vi "Get Command and Process.vi"(8 "Error In":errorcluster, 10 "FPGA Ref":T3, 11 "Network Info":T1 {"Last Comm Time" format="%<%H:%M:%S%3u\n%Y/%m/%d>T"; "Remote Port" format="%.0x"}) -> (0 "Error Out":errorcluster, 2 "Connection Dormant":bool, 3 "Network Info out":T1 {"Last Comm Time" format="%<%H:%M:%S%3u\n%Y/%m/%d>T"; "Remote Port" format="%.0x"})   [LabVIEW 2020]
doc: "Author: Scott Hannahs <sth@magnet.fsu.edu>\nCopyright 2018 Florida State University, All rights reserved."
uses:
  RT Controls/Network Info.ctl
  RT Controls/RT System Auth Level.ctl
  RT Controls/FPGA SCH Digitizer Ref.ctl
  Init Coil Calibration/FPGA Magnet Config.ctl
  SCH Data Controls/SCH Data 2 RT.ctl
  RT Host Globals.vi
  TCP Functions/TCP Write Length and Data (STR).vi
  TCP Functions/TCP Write Length and Data (DBL).vi
  TCP Functions/TCP Write Length and Data (2D Array DBL).vi
  TCP Functions/TCP Read Length and Value (STR).vi
  TCP Functions/TCP Read Length and Value (Array Dbl).vi
  <vilib>/Utility/error.llb/Error Cluster From Error Code.vi
  <vilib>/rvi/errors/niLvFpgaAdjustHostInterfaceError.vi
  TCP Functions/TCP Read Length and Value (Double).vi
  TCP Functions/TCP Read Length and Value (U32).vi
  TCP Functions/TCP Read Length and Value (I16).vi
  TCP Functions/TCP Read Length and Value (Bool).vi
  TCP Functions/TCP Read Length and Value (I32).vi
  TCP Functions/TCP Read Length and Value (U16).vi
  TCP Functions/TCP Write Length and Data (Array DBL).vi
  TCP Functions/TCP Write Length and Data (U32).vi
  TCP Functions/TCP Write Length and Data (Bool).vi
  TCP Functions/TCP Write Length and Data (I16).vi
  TCP Functions/TCP Write Length and Data (I32).vi
  TCP Functions/TCP Write Length and Data (Array I16).vi
  TCP Functions/TCP Write Length and Data (U16).vi
  TCP Functions/TCP Write Length and Data (DateStamp).vi
  TCP Functions/TCP Write Length and Data (Array Str).vi
  <vilib>/rvi/interface/nirviReadWriteControl/nirviReadWriteControl.xnode
  NiFpgaLv.dll
  <vilib>/rvi/interface/Simulation/niFpgaSimulationCallBeginRW.vi
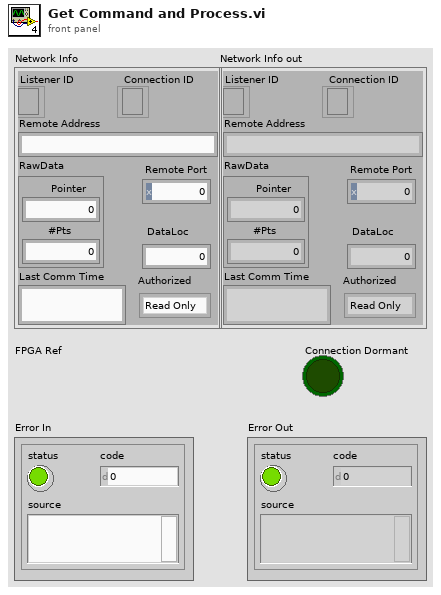
[diagram p1: front panel]
types:
  T1 = typedef "Network Info.ctl" = cluster{"Listener ID":refnum<k5>, "Connection ID":refnum<k5>, "Remote Address":string, "Remote Port":u16, "DataLoc":u32, "RawData":cluster{"#Pts":u32, "Pointer":u32}, "Last Comm Time":timestamp, "Authorized":T2}
  T2 = typedef "RT System Auth Level.ctl" = enum16{"Read Only", "Operator", "Admin"}
  T3 = typedef "FPGA SCH Digitizer Ref.ctl" = refnum<k20>
  T4 = typedef "FPGA Magnet Config.ctl" = cluster{"#Coils":u32, "Coil Inductances":T5[], "Max Coil Currents":T5[], "Max Coil Volt Dev":T5[], "Coil A Coefficients":T5[], "Coil B Coefficients":T5[], "Coil C Coefficients":T5[], "Coil D Coefficients":T5[], "Max Coil Temp":T5[], " Pressure Range":T5[], "Temp Coef":T5[], "Offsets":T5[], "Scale Factors":T5[]}
  T5 = typedef "SCH Data 2 RT.ctl" = fxp<+/-,38,12>
  T6 = enum16{"Input Voltage", "Zero Voltage", "Calibrate Voltage"}
  T7 = typedef "FPGA Configure Parameters.ctl" = cluster{"Ln2 Filter Size":i16, "VT Quench Tick Limit":u32, "VT Quench Volt Limit":dbl, "Joint Tick Limit":u32, "Joint Volt Limit":dbl, "CoWound Volt Limit":dbl, "CoWound Tick Limit":u32, "SC Bus Limit":dbl, "SC Bus Tick Limit":u32, "ResMag Tick Limit":u32, "DAQ Cycle Ticks":u32, "Res Mag dI/dt Delay":u32, "dI/dT scaling":dbl, "Pressure Inlet Limit (BarA)":dbl, "Bore Tube Volt Limit":dbl, "Pressure Outlet Limit (BarA)":dbl, "Activation Current (kA)":dbl, "Dump Resistor Scale Factor":dbl, "Co-Wound Asymmetry Factor":dbl, "Co-Wound Scale Factor":dbl, "Layer Scale Factors":dbl[], "Fudge Factors":dbl[], "Joint Scale Factors":dbl[], "SC Bus Scale":dbl[], "Pressure Scale Factor":dbl[], "# Consecutive Zeros Fault":i16, "Digitize Convert Ticks":u32, "Digitize Reset Ticks":u32, "Convert Clock Ticks":u32, "Digitize Read Delay Ticks":u32, "Digitize # Bits":u32, "HTS Lead Tick Limit":u32, "Res Lead Tick Limit":u32, "HTS Lead Trip":dbl, "Res Lead Limit":dbl, "HTS Lead FRZ":dbl, "HTS Lead Warn":dbl, "Low Current (kA)":dbl, "Low Current Ticks":u32, "Low Current Delay Factor":u16, "HTS Resistance (nOhm)":dbl[], "Ticks to Close Relief":u32, "All Breaker Tick Limit":u32, "HTS Offset (microV)":dbl[], "Delay Ticks Between Bkr Reset":u32, "Breaker Reset Ticks":u32, "PS Enable Reset Ticks":u32, "Reset Digitizer Ticks":u32, "Pressure Inlet Cooldown Limit":dbl, "Pressure Outlet Cooldown Limit":dbl, "Notification Email":string}
  T8 = cluster{"#Coils":u32, "Coil Inductances":fxp<+/-,38,12>[], "Max Coil Currents":fxp<+/-,38,12>[], "Max Coil Volt Dev":fxp<+/-,38,12>[], "Coil A Coefficients":fxp<+/-,38,12>[], "Coil B Coefficients":fxp<+/-,38,12>[], "Coil C Coefficients":fxp<+/-,38,12>[], "Coil D Coefficients":fxp<+/-,38,12>[], "Max Coil Temp":fxp<+/-,38,12>[], " Pressure Range":fxp<+/-,38,12>[], "Temp Coef":fxp<+/-,38,12>[], "Offsets":fxp<+/-,38,12>[], "Scale Factors":fxp<+/-,38,12>[]}
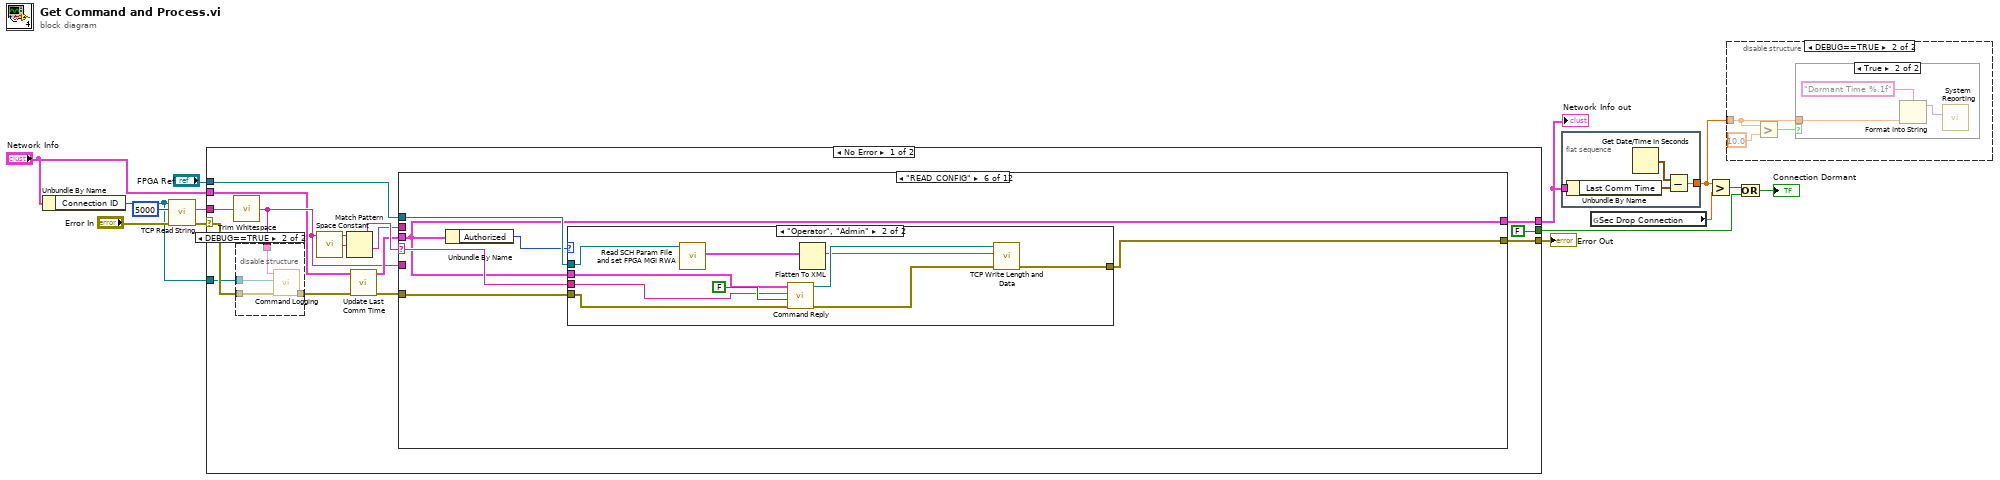
[diagram p0: block diagram]
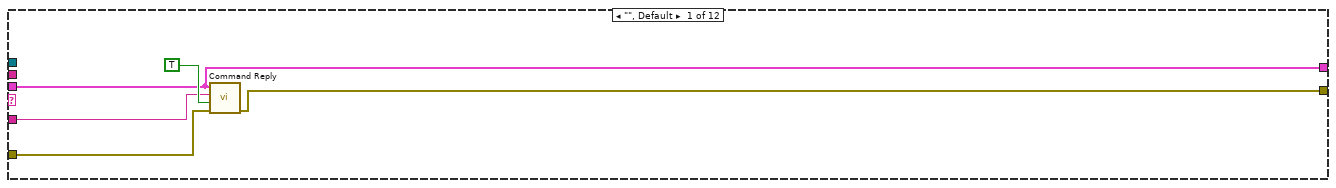
[diagram p5: hidden frame]
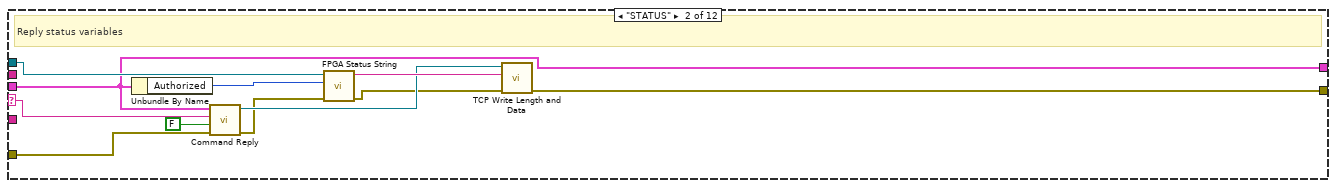
[diagram p6: hidden frame]
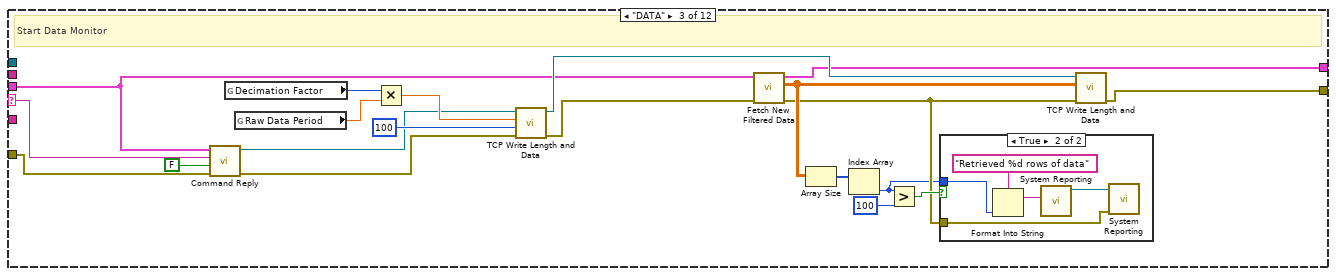
[diagram p7: hidden frame]
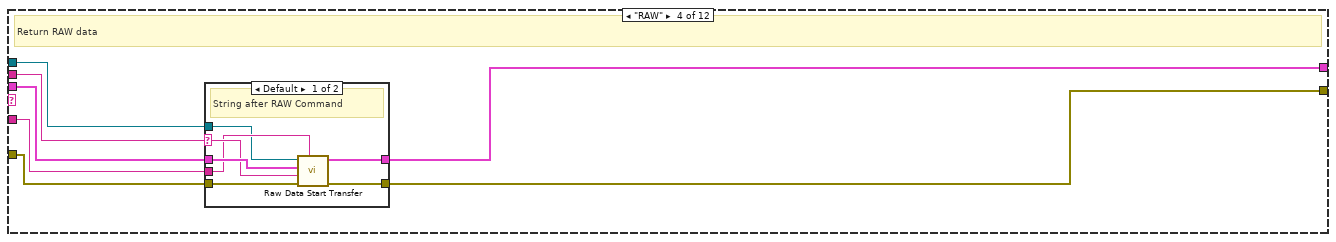
[diagram p9: hidden frame]
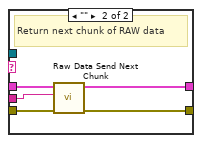
[diagram p10: hidden frame]
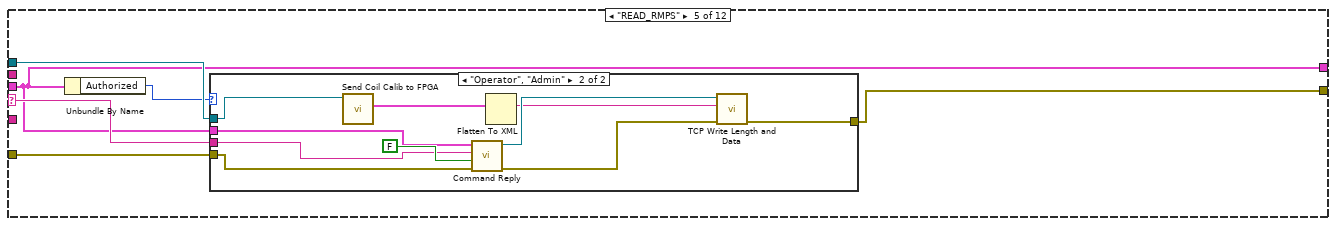
[diagram p11: hidden frame]
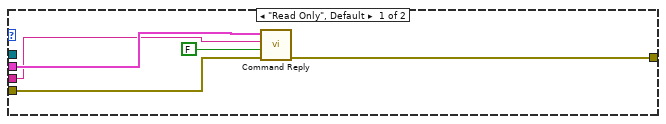
[diagram p12: hidden frame]
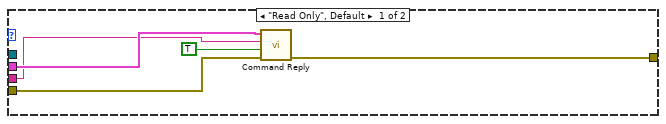
[diagram p13: hidden frame]
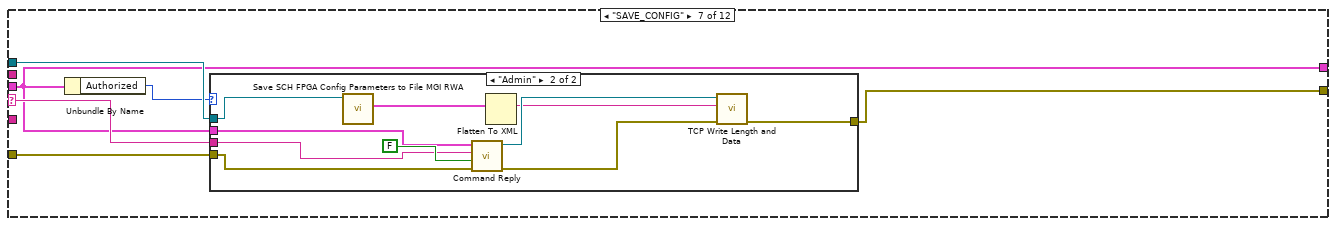
[diagram p14: hidden frame]
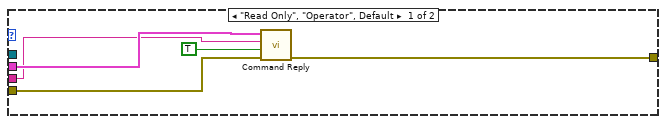
[diagram p15: hidden frame]
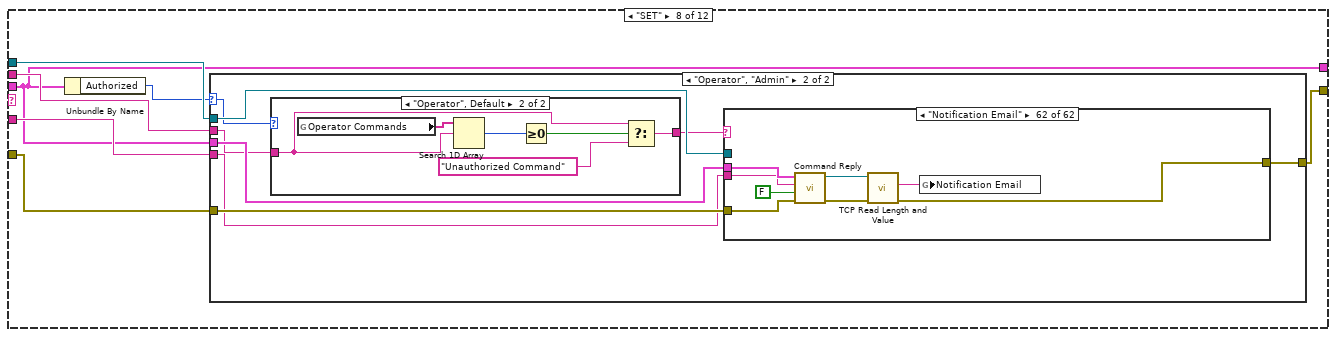
[diagram p16: hidden frame]
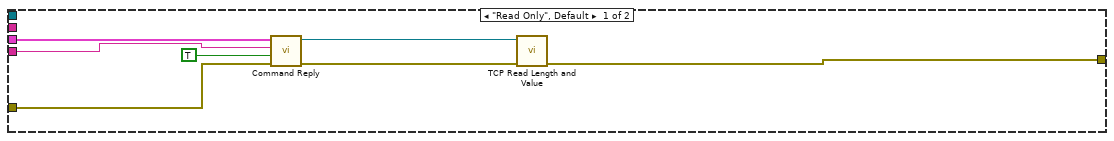
[diagram p17: hidden frame]
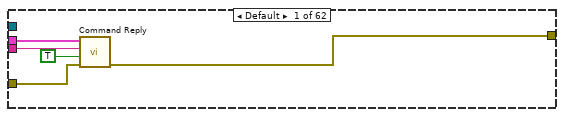
[diagram p19: hidden frame]
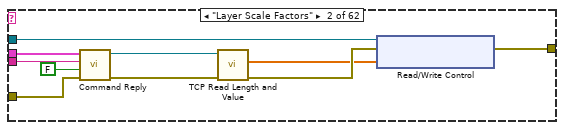
[diagram p20: hidden frame]
diagram:
  n1 = Unbundle By Name("Network Info") -> ("Connection ID"=w3:refnum<k5>)
  n2 = call "TCP Read String.vi"("Error In"="Error In", "timeout ms (1000)"=5000 ("timeout ms (25000)"), "TCP Network Connection in"=w3) -> ("Error Out"=w11:errorcluster, "String"=w9:string)  [unwired: 6 in, 1 out]
  n3 = case shown="No Error" w11 {
    selector: w11 -> [w21 w1545]
    tunnel: "Network Info" -> [w16 w1547]
    tunnel: w9 -> [w19 _]
    tunnel: "FPGA Ref" -> [w29 _]
    tunnel: [w28 w1548] -> w13
    tunnel: [w22 w1547] -> w7
    tunnel: [FALSE ("specific error cleared?") w1540] -> w4
    tunnel: w3 -> [w15 _]
    frame No Error {
      n4 = call <vilib>:"Trim Whitespace.vi"("string"=w19) -> ("trimmed string"=w17:string)  [unwired: 1 in]
      n5 = disable-structure shown="DEBUG==TRUE" {
        disable-tunnel: w21 -> [w30 w34]
        disable-tunnel: [w30 w33] -> w20
        disable-tunnel: w17 -> [_ w32]
        disable-tunnel: w15 -> [_ w31]
        frame condition #0 (active) {
        }
        frame condition #1 {
          n6 = call "Command Logging.vi"("error in (no error)"=w34, "TCP Network Connection in"=w31, "String"=w32) -> ("error out"=w33:errorcluster)  [unwired: 8 in]
        }
      }
      n7 = call <vilib>:"Space Constant.vi"() -> ("String"=w26:string)
      n8 = Match Pattern(string=w17, regular expression=w26) -> (before substring=w27:string, after substring=w25:string)  [unwired: 1 in, 2 out]
      n9 = call "Update Last Comm Time.vi"("error in (no error)"=w20, "Network Info in"=w16) -> ("error out"=w24:errorcluster, "Network Info out"=w23:T1)  [unwired: 8 in]
      n10 = case shown="\"READ_CONFIG\"" w27 {
        selector: w27 -> [_ w42 w62 _ w99 w121 w142 _ _ w1503 _ _]
        tunnel: w23 -> [w35 w41 w59 w77 w95 w116 w137 w158 w812 w1500 w1511 w1527]
        tunnel: w29 -> [_ w50 _ w78 w100 w120 w141 w164 w817 _ _ _]
        tunnel: w24 -> [w38 w44 w70 w82 w98 w119 w140 w163 w816 w1505 w1518 w1532]
        tunnel: [w37 w43 w61 w81 w97 w118 w139 w162 w815 w1506 w1515 w1523] -> w28
        tunnel: w25 -> [_ _ _ w80 _ _ _ w161 w814 _ w1514 _]
        tunnel: w17 -> [w36 _ _ w79 _ _ _ w160 w813 _ w1513 w1529]
        tunnel: [w35 w41 w58 w76 w95 w116 w137 w158 w812 w1500 w1511 w1519] -> w22
        frame "", Default {
          n11 = call "Command Reply.vi"("Error In"=w38, "Error?"=TRUE ("s"), "String"=w36, "Network Info"=w35) -> ("error out"=w37:errorcluster)  [unwired: 6 in, 1 out]
        }
        frame "STATUS" {
          # "Reply status variables"
          n12 = Unbundle By Name(w41) -> ("Authorized"=w40:T2)
          n13 = call "Command Reply.vi"("Error In"=w44, "Error?"=FALSE, "String"=w42, "Network Info"=w41) -> ("error out"=w46:errorcluster, "TCP Network Connection out"=w48:refnum<k5>)  [unwired: 6 in]
          n14 = call "FPGA Status String.vi"("error in (no error)"=w46, "Authorized"=w40, "Refnum in"=w50) -> ("error out"=w45:errorcluster, "Data String"=w49:string)  [unwired: 7 in]
          n15 = call-poly "TCP Write Length and Data.vi"("Error In"=w45, "Data"=w49, "connection ID"=w48) -> ("Error Out"=w43:errorcluster)  [unwired: 7 in, 1 out]
        }
        frame "DATA" {
          # "Start Data Monitor"
          n16 = call "Command Reply.vi"("Error In"=w70, "Error?"=FALSE, "String"=w62, "Network Info"=w59) -> ("error out"=w64:errorcluster, "TCP Network Connection out"=w65:refnum<k5>)  [unwired: 6 in]
          n17 = global read "RT Host Globals.vi" "Decimation Factor"() -> (w67:u32)
          n18 = global read "RT Host Globals.vi" "Raw Data Period"() -> (w66:dbl)
          n19 = Multiply(x=w67, y=w66) -> (x*y=w68:dbl)
          n20 = call-poly "TCP Write Length and Data.vi"("Error In"=w64, "Timeout"=100, "Data"=w68, "connection ID"=w65) -> ("Error Out"=w57:errorcluster, "connection ID out"=w60:refnum<k5>)  [unwired: 6 in]
          n21 = call "Fetch New Filtered Data.vi"("error in (no error)"=w57, "Network Info in"=w59) -> ("error out"=w52:errorcluster, "Data Out"=w55:dbl[][], "Network Info Out"=w58:T1)  [unwired: 6 in]
          n22 = Array Size(array=w55) -> (size(s)=w56:i32[])
          n23 = Index Array(array=w56) -> (element=w51:i32)  [unwired: 1 in]
          n24 = Greater?(x=w51, y=100) -> (0:w53:bool)
          n25 = case shown="True" w53 {
            tunnel: w52 -> [_ w73]
            tunnel: w51 -> [_ w75]
            frame False {
            }
            frame True {
              n26 = Format Into String(format string="Retrieved %d rows of data", w75) -> (resulting string=w72:string)  [unwired: 2 in, 1 out]
              n27 = call "System Reporting.vi"("String"=w72) -> ("Byte Stream File out"=w71:refnum<file>)  [unwired: 9 in, 1 out]
              n28 = call "System Reporting.vi"("Error In"=w73, "Byte Stream File in"=w71) -> ()  [unwired: 8 in, 2 out]
            }
          }
          n29 = call-poly "TCP Write Length and Data.vi"("Error In"=w52, "Data"=w55, "connection ID"=w60) -> ("Error Out"=w61:errorcluster)  [unwired: 7 in, 1 out]
        }
        frame "RAW" {
          # "Return RAW data"
          n30 = case shown="Default" w80 {
            selector: w80 -> [w87 _]
            tunnel: w77 -> [w88 w94]
            tunnel: w79 -> [w86 w93]
            tunnel: w82 -> [w85 w92]
            tunnel: [w89 w91] -> w81
            tunnel: w78 -> [w84 _]
            tunnel: [w83 w90] -> w76
            frame Default {
              # "String after RAW Command"
              n31 = call "Raw Data Start Transfer.vi"("Command string"=w86, "error in (no error)"=w85, "#pts string"=w87, "Network Info"=w88, "Refnum in"=w84) -> ("error out"=w89:errorcluster, "Network Info Out"=w83:T1)  [unwired: 5 in]
            }
            frame "" {
              # "Return next chunk of RAW data"
              n32 = call "Raw Data Send Next Chunk.vi"("error in (no error)"=w92, "trimmed string"=w93, "Network Info"=w94) -> ("error out"=w91:errorcluster, "Network Info Out"=w90:T1)  [unwired: 7 in]
            }
          }
        }
        frame "READ_RMPS" {
          n33 = Unbundle By Name(w95) -> ("Authorized"=w96:T2)
          n34 = case shown="\"Operator\", \"Admin\"" w96 {
            tunnel: w100 -> [_ w115]
            tunnel: w95 -> [w104 w113]
            tunnel: w99 -> [w103 w112]
            tunnel: w98 -> [w102 w107]
            tunnel: [w101 w106] -> w97
            frame "Read Only", Default {
              n35 = call "Command Reply.vi"("Error In"=w102, "Error?"=FALSE, "String"=w103, "Network Info"=w104) -> ("error out"=w101:errorcluster)  [unwired: 6 in, 1 out]
            }
            frame "Operator", "Admin" {
              n36 = call "Send Coil Calib to FPGA.vi"("Refnum in"=w115) -> ("Magnet Configuration Data"=w111:T4)  [unwired: 8 in, 2 out]
              n37 = call "Command Reply.vi"("Error In"=w107, "Error?"=FALSE, "String"=w112, "Network Info"=w113) -> ("error out"=w108:errorcluster, "TCP Network Connection out"=w110:refnum<k5>)  [unwired: 6 in]
              n38 = Flatten To XML(6:w111) -> (2:w109:string)
              n39 = call-poly "TCP Write Length and Data.vi"("Error In"=w108, "Data"=w109, "connection ID"=w110) -> ("Error Out"=w106:errorcluster)  [unwired: 7 in, 1 out]
            }
          }
        }
        frame "READ_CONFIG" {
          n40 = Unbundle By Name(w116) -> ("Authorized"=w117:T2)
          n41 = case shown="\"Operator\", \"Admin\"" w117 {
            tunnel: w116 -> [w126 w135]
            tunnel: w121 -> [w125 w134]
            tunnel: w120 -> [_ w130]
            tunnel: w119 -> [w123 w128]
            tunnel: [w122 w127] -> w118
            frame "Read Only", Default {
              n42 = call "Command Reply.vi"("Error In"=w123, "Error?"=TRUE, "String"=w125, "Network Info"=w126) -> ("error out"=w122:errorcluster)  [unwired: 6 in, 1 out]
            }
            frame "Operator", "Admin" {
              n43 = call "Read SCH Param File and set FPGA MGI RWA.vi"("FPGA Refnum in"=w130) -> ("FPGA Configuration Values"=w129:T7)  [unwired: 8 in, 2 out]
              n44 = call "Command Reply.vi"("Error In"=w128, "Error?"=FALSE, "String"=w134, "Network Info"=w135) -> ("error out"=w131:errorcluster, "TCP Network Connection out"=w133:refnum<k5>)  [unwired: 6 in]
              n45 = Flatten To XML(6:w129) -> (2:w132:string)
              n46 = call-poly "TCP Write Length and Data.vi"("Error In"=w131, "Data"=w132, "connection ID"=w133) -> ("Error Out"=w127:errorcluster)  [unwired: 7 in, 1 out]
            }
          }
        }
        frame "SAVE_CONFIG" {
          n47 = Unbundle By Name(w137) -> ("Authorized"=w138:T2)
          n48 = case shown="\"Admin\"" w138 {
            tunnel: w137 -> [w146 w156]
            tunnel: w142 -> [w145 w155]
            tunnel: w141 -> [_ w152]
            tunnel: w140 -> [w144 w149]
            tunnel: [w143 w148] -> w139
            frame "Read Only", "Operator", Default {
              n49 = call "Command Reply.vi"("Error In"=w144, "Error?"=TRUE, "String"=w145, "Network Info"=w146) -> ("error out"=w143:errorcluster)  [unwired: 6 in, 1 out]
            }
            frame "Admin" {
              n50 = call "Save SCH FPGA Config Parameters to File MGI RWA.vi"("Refnum in"=w152) -> ("FPGA Configuration Values"=w150:T7)  [unwired: 8 in, 2 out]
              n51 = call "Command Reply.vi"("Error In"=w149, "Error?"=FALSE, "String"=w155, "Network Info"=w156) -> ("error out"=w151:errorcluster, "TCP Network Connection out"=w154:refnum<k5>)  [unwired: 6 in]
              n52 = Flatten To XML(6:w150) -> (2:w153:string)
              n53 = call-poly "TCP Write Length and Data.vi"("Error In"=w151, "Data"=w153, "connection ID"=w154) -> ("Error Out"=w148:errorcluster)  [unwired: 7 in, 1 out]
            }
          }
        }
        frame "SET" {
          n54 = Unbundle By Name(w158) -> ("Authorized"=w159:T2)
          n55 = case shown="\"Operator\", \"Admin\"" w159 {
            selector: w159 -> [_ w174]
            tunnel: w164 -> [_ w179]
            tunnel: w163 -> [w167 w178]
            tunnel: [w168 w177] -> w162
            tunnel: w161 -> [_ w173]
            tunnel: w160 -> [w166 w176]
            tunnel: w158 -> [w165 w175]
            frame "Read Only", Default {
              n56 = call "Command Reply.vi"("Error In"=w167, "Error?"=TRUE, "String"=w166, "Network Info"=w165) -> ("error out"=w171:errorcluster, "TCP Network Connection out"=w170:refnum<k5>)  [unwired: 6 in]
              n57 = call-poly "TCP Read Length and Value.vi"("error in (no error)"=w171, "TCP Network Connection in"=w170) -> ("error out"=w168:errorcluster)  [unwired: 7 in, 2 out]
            }
            frame "Operator", "Admin" {
              n58 = case shown="\"Operator\", Default" w174 {
                tunnel: [w180 w182] -> w172
                tunnel: w173 -> [w180 w183]
                frame "Admin" {
                }
                frame "Operator", Default {
                  n59 = global read "RT Host Globals.vi" "Operator Commands"() -> (w186:string[])
                  n60 = Search 1D Array(1D array=w186, element=w183) -> (index of element=w185:i32)  [unwired: 1 in]
                  n61 = Greater Or Equal To 0?(x=w185) -> (x >= 0?=w184:bool)
                  n62 = Select(t=w183, s=w184, f="Unauthorized Command") -> (s? t:f=w182:string)
                }
              }
              n63 = case shown="\"Notification Email\"" w172 {
                tunnel: w176 -> [w191 w199 w209 w219 w229 w239 w249 w259 w269 w279 w289 w299 w309 w319 w329 w339 w349 w359 w369 w379 w389 w399 w409 w419 w429 w439 w449 w459 w469 w479 w489 w499 w509 w519 w529 w539 w549 w559 w569 w579 w589 w599 w609 w619 w633 w643 w653 w663 w673 w683 w693 w703 w713 w723 w733 w743 w755 w765 w775 w785 w795 w809]
                tunnel: w175 -> [w190 w200 w210 w220 w230 w240 w250 w260 w270 w280 w290 w300 w310 w320 w330 w340 w350 w360 w370 w380 w390 w400 w410 w420 w430 w440 w450 w460 w470 w480 w490 w500 w510 w520 w530 w540 w550 w560 w570 w580 w590 w600 w610 w620 w634 w644 w654 w664 w674 w684 w694 w704 w714 w724 w734 w744 w756 w766 w776 w786 w796 w810]
                tunnel: w179 -> [_ w196 w206 w216 w226 w236 w246 w256 w266 w276 w286 w296 w306 w316 w326 w336 w346 w356 w366 w376 w386 w396 w406 w416 w426 w436 w446 w456 w466 w476 w486 w496 w506 w516 w526 w536 w546 w556 w566 w576 w586 w596 w606 w616 w630 w639 w650 w660 w670 w680 w690 w700 w710 w720 w730 w740 w749 w760 w770 w780 w792 _]
                tunnel: w178 -> [w188 w193 w203 w213 w223 w233 w243 w253 w263 w273 w283 w293 w303 w313 w323 w333 w343 w353 w364 w375 w384 w395 w404 w414 w424 w434 w444 w453 w463 w474 w484 w494 w504 w514 w524 w534 w543 w553 w563 w573 w583 w593 w603 w614 w629 w640 w649 w659 w669 w679 w689 w699 w709 w719 w729 w739 w752 w762 w772 w782 w790 w806]
                tunnel: [w187 w192 w202 w212 w222 w232 w242 w252 w262 w272 w282 w292 w302 w312 w322 w332 w342 w352 w363 w374 w383 w394 w403 w413 w423 w433 w443 w452 w462 w473 w483 w493 w503 w513 w523 w533 w542 w552 w562 w572 w582 w592 w602 w613 w628 w636 w648 w658 w668 w678 w688 w698 w708 w718 w728 w738 w751 w758 w768 w778 w789 w805] -> w177
                frame Default {
                  n64 = call "Command Reply.vi"("Error In"=w188, "Error?"=TRUE, "String"=w191, "Network Info"=w190) -> ("error out"=w187:errorcluster)  [unwired: 6 in, 1 out]
                }
                frame "Layer Scale Factors" {
                  n65 = call "Command Reply.vi"("Error In"=w193, "Error?"=FALSE, "String"=w199, "Network Info"=w200) -> ("error out"=w197:errorcluster, "TCP Network Connection out"=w198:refnum<k5>)  [unwired: 6 in]
                  n66 = call-poly "TCP Read Length and Value.vi"("error in (no error)"=w197, "TCP Network Connection in"=w198) -> ("error out"=w195:errorcluster, "Output"=w194:dbl[])  [unwired: 7 in, 1 out]
                  n67 = xnode "Read/Write Control"("FPGA VI Reference In"=w196, "error in"=w195, "Layer Scale Factors"=w194) -> ("error out"=w192:errorcluster)  [unwired: 1 out]
                }
                frame "Fudge Factors" {
                  n68 = call "Command Reply.vi"("Error In"=w203, "Error?"=FALSE, "String"=w209, "Network Info"=w210) -> ("error out"=w207:errorcluster, "TCP Network Connection out"=w208:refnum<k5>)  [unwired: 6 in]
                  n69 = call-poly "TCP Read Length and Value.vi"("error in (no error)"=w207, "TCP Network Connection in"=w208) -> ("error out"=w205:errorcluster, "Output"=w204:dbl[])  [unwired: 7 in, 1 out]
                  n70 = xnode "Read/Write Control"("FPGA VI Reference In"=w206, "error in"=w205, "Fudge Factors"=w204) -> ("error out"=w202:errorcluster)  [unwired: 1 out]
                }
                frame "Co-Wound Scale Factor" {
                  n71 = call "Command Reply.vi"("Error In"=w213, "Error?"=FALSE, "String"=w219, "Network Info"=w220) -> ("error out"=w217:errorcluster, "TCP Network Connection out"=w218:refnum<k5>)  [unwired: 6 in]
                  n72 = call-poly "TCP Read Length and Value.vi"("error in (no error)"=w217, "TCP Network Connection in"=w218) -> ("error out"=w215:errorcluster, "Output"=w214:dbl)  [unwired: 7 in, 1 out]
                  n73 = xnode "Read/Write Control"("FPGA VI Reference In"=w216, "error in"=w215, "Co-Wound Scale Factor"=w214) -> ("error out"=w212:errorcluster)  [unwired: 1 out]
                }
                frame "Co-Wound Asymmetry Factor" {
                  n74 = call "Command Reply.vi"("Error In"=w223, "Error?"=FALSE, "String"=w229, "Network Info"=w230) -> ("error out"=w227:errorcluster, "TCP Network Connection out"=w228:refnum<k5>)  [unwired: 6 in]
                  n75 = call-poly "TCP Read Length and Value.vi"("error in (no error)"=w227, "TCP Network Connection in"=w228) -> ("error out"=w225:errorcluster, "Output"=w224:dbl)  [unwired: 7 in, 1 out]
                  n76 = xnode "Read/Write Control"("FPGA VI Reference In"=w226, "error in"=w225, "Co-Wound Asymmetry Factor"=w224) -> ("error out"=w222:errorcluster)  [unwired: 1 out]
                }
                frame "Dump Resistor Scale Factor" {
                  n77 = call "Command Reply.vi"("Error In"=w233, "Error?"=FALSE, "String"=w239, "Network Info"=w240) -> ("error out"=w237:errorcluster, "TCP Network Connection out"=w238:refnum<k5>)  [unwired: 6 in]
                  n78 = call-poly "TCP Read Length and Value.vi"("error in (no error)"=w237, "TCP Network Connection in"=w238) -> ("error out"=w235:errorcluster, "Output"=w234:dbl)  [unwired: 7 in, 1 out]
                  n79 = xnode "Read/Write Control"("FPGA VI Reference In"=w236, "error in"=w235, "Dump Resistor Scale Factor"=w234) -> ("error out"=w232:errorcluster)  [unwired: 1 out]
                }
                frame "Joint Scale Factors" {
                  n80 = call "Command Reply.vi"("Error In"=w243, "Error?"=FALSE, "String"=w249, "Network Info"=w250) -> ("error out"=w247:errorcluster, "TCP Network Connection out"=w248:refnum<k5>)  [unwired: 6 in]
                  n81 = call-poly "TCP Read Length and Value.vi"("error in (no error)"=w247, "TCP Network Connection in"=w248) -> ("error out"=w245:errorcluster, "Output"=w244:dbl[])  [unwired: 7 in, 1 out]
                  n82 = xnode "Read/Write Control"("FPGA VI Reference In"=w246, "error in"=w245, "Joint Scale Factors"=w244) -> ("error out"=w242:errorcluster)  [unwired: 1 out]
                }
                frame "SC Bus Scale" {
                  n83 = call "Command Reply.vi"("Error In"=w253, "Error?"=FALSE, "String"=w259, "Network Info"=w260) -> ("error out"=w257:errorcluster, "TCP Network Connection out"=w258:refnum<k5>)  [unwired: 6 in]
                  n84 = call-poly "TCP Read Length and Value.vi"("error in (no error)"=w257, "TCP Network Connection in"=w258) -> ("error out"=w255:errorcluster, "Output"=w254:dbl[])  [unwired: 7 in, 1 out]
                  n85 = xnode "Read/Write Control"("FPGA VI Reference In"=w256, "error in"=w255, "SC Bus Scale"=w254) -> ("error out"=w252:errorcluster)  [unwired: 1 out]
                }
                frame "HTS Resistance (nOhm)" {
                  n86 = call "Command Reply.vi"("Error In"=w263, "Error?"=FALSE, "String"=w269, "Network Info"=w270) -> ("error out"=w267:errorcluster, "TCP Network Connection out"=w268:refnum<k5>)  [unwired: 6 in]
                  n87 = call-poly "TCP Read Length and Value.vi"("error in (no error)"=w267, "TCP Network Connection in"=w268) -> ("error out"=w265:errorcluster, "Output"=w264:dbl[])  [unwired: 7 in, 1 out]
                  n88 = xnode "Read/Write Control"("FPGA VI Reference In"=w266, "error in"=w265, "HTS Resistance (nOhm)"=w264) -> ("error out"=w262:errorcluster)  [unwired: 1 out]
                }
                frame "HTS Offset (microV)" {
                  n89 = call "Command Reply.vi"("Error In"=w273, "Error?"=FALSE, "String"=w279, "Network Info"=w280) -> ("error out"=w277:errorcluster, "TCP Network Connection out"=w278:refnum<k5>)  [unwired: 6 in]
                  n90 = call-poly "TCP Read Length and Value.vi"("error in (no error)"=w277, "TCP Network Connection in"=w278) -> ("error out"=w275:errorcluster, "Output"=w274:dbl[])  [unwired: 7 in, 1 out]
                  n91 = xnode "Read/Write Control"("FPGA VI Reference In"=w276, "error in"=w275, "HTS Offset (microV)"=w274) -> ("error out"=w272:errorcluster)  [unwired: 1 out]
                }
                frame "Pressure Scale Factor" {
                  n92 = call "Command Reply.vi"("Error In"=w283, "Error?"=FALSE, "String"=w289, "Network Info"=w290) -> ("error out"=w287:errorcluster, "TCP Network Connection out"=w288:refnum<k5>)  [unwired: 6 in]
                  n93 = call-poly "TCP Read Length and Value.vi"("error in (no error)"=w287, "TCP Network Connection in"=w288) -> ("error out"=w285:errorcluster, "Output"=w284:dbl[])  [unwired: 7 in, 1 out]
                  n94 = xnode "Read/Write Control"("FPGA VI Reference In"=w286, "error in"=w285, "Pressure Scale Factor"=w284) -> ("error out"=w282:errorcluster)  [unwired: 1 out]
                }
                frame "VT Quench Tick Limit" {
                  n95 = call "Command Reply.vi"("Error In"=w293, "Error?"=FALSE, "String"=w299, "Network Info"=w300) -> ("error out"=w297:errorcluster, "TCP Network Connection out"=w298:refnum<k5>)  [unwired: 6 in]
                  n96 = call-poly "TCP Read Length and Value.vi"("error in (no error)"=w297, "TCP Network Connection in"=w298) -> ("error out"=w295:errorcluster, "Output"=w294:u32)  [unwired: 7 in, 1 out]
                  n97 = xnode "Read/Write Control"("FPGA VI Reference In"=w296, "error in"=w295, "VT Quench Tick Limit"=w294) -> ("error out"=w292:errorcluster)  [unwired: 1 out]
                }
                frame "Joint Tick Limit" {
                  n98 = call "Command Reply.vi"("Error In"=w303, "Error?"=FALSE, "String"=w309, "Network Info"=w310) -> ("error out"=w307:errorcluster, "TCP Network Connection out"=w308:refnum<k5>)  [unwired: 6 in]
                  n99 = call-poly "TCP Read Length and Value.vi"("error in (no error)"=w307, "TCP Network Connection in"=w308) -> ("error out"=w305:errorcluster, "Output"=w304:u32)  [unwired: 7 in, 1 out]
                  n100 = xnode "Read/Write Control"("FPGA VI Reference In"=w306, "error in"=w305, "Joint Tick Limit"=w304) -> ("error out"=w302:errorcluster)  [unwired: 1 out]
                }
                frame "CoWound Tick Limit" {
                  n101 = call "Command Reply.vi"("Error In"=w313, "Error?"=FALSE, "String"=w319, "Network Info"=w320) -> ("error out"=w317:errorcluster, "TCP Network Connection out"=w318:refnum<k5>)  [unwired: 6 in]
                  n102 = call-poly "TCP Read Length and Value.vi"("error in (no error)"=w317, "TCP Network Connection in"=w318) -> ("error out"=w315:errorcluster, "Output"=w314:u32)  [unwired: 7 in, 1 out]
                  n103 = xnode "Read/Write Control"("FPGA VI Reference In"=w316, "error in"=w315, "CoWound Tick Limit"=w314) -> ("error out"=w312:errorcluster)  [unwired: 1 out]
                }
                frame "SC Bus Tick Limit" {
                  n104 = call "Command Reply.vi"("Error In"=w323, "Error?"=FALSE, "String"=w329, "Network Info"=w330) -> ("error out"=w327:errorcluster, "TCP Network Connection out"=w328:refnum<k5>)  [unwired: 6 in]
                  n105 = call-poly "TCP Read Length and Value.vi"("error in (no error)"=w327, "TCP Network Connection in"=w328) -> ("error out"=w325:errorcluster, "Output"=w324:u32)  [unwired: 7 in, 1 out]
                  n106 = xnode "Read/Write Control"("FPGA VI Reference In"=w326, "error in"=w325, "SC Bus Tick Limit"=w324) -> ("error out"=w322:errorcluster)  [unwired: 1 out]
                }
                frame "HTS Lead Tick Limit" {
                  n107 = call "Command Reply.vi"("Error In"=w333, "Error?"=FALSE, "String"=w339, "Network Info"=w340) -> ("error out"=w337:errorcluster, "TCP Network Connection out"=w338:refnum<k5>)  [unwired: 6 in]
                  n108 = call-poly "TCP Read Length and Value.vi"("error in (no error)"=w337, "TCP Network Connection in"=w338) -> ("error out"=w335:errorcluster, "Output"=w334:u32)  [unwired: 7 in, 1 out]
                  n109 = xnode "Read/Write Control"("FPGA VI Reference In"=w336, "error in"=w335, "HTS Lead Tick Limit"=w334) -> ("error out"=w332:errorcluster)  [unwired: 1 out]
                }
                frame "Res Lead Tick Limit" {
                  n110 = call "Command Reply.vi"("Error In"=w343, "Error?"=FALSE, "String"=w349, "Network Info"=w350) -> ("error out"=w347:errorcluster, "TCP Network Connection out"=w348:refnum<k5>)  [unwired: 6 in]
                  n111 = call-poly "TCP Read Length and Value.vi"("error in (no error)"=w347, "TCP Network Connection in"=w348) -> ("error out"=w345:errorcluster, "Output"=w344:u32)  [unwired: 7 in, 1 out]
                  n112 = xnode "Read/Write Control"("FPGA VI Reference In"=w346, "error in"=w345, "Res Lead Tick Limit"=w344) -> ("error out"=w342:errorcluster)  [unwired: 1 out]
                }
                frame "ResMag Tick Limit" {
                  n113 = call "Command Reply.vi"("Error In"=w353, "Error?"=FALSE, "String"=w359, "Network Info"=w360) -> ("error out"=w357:errorcluster, "TCP Network Connection out"=w358:refnum<k5>)  [unwired: 6 in]
                  n114 = call-poly "TCP Read Length and Value.vi"("error in (no error)"=w357, "TCP Network Connection in"=w358) -> ("error out"=w355:errorcluster, "Output"=w354:u32)  [unwired: 7 in, 1 out]
                  n115 = xnode "Read/Write Control"("FPGA VI Reference In"=w356, "error in"=w355, "ResMag Tick Limit"=w354) -> ("error out"=w352:errorcluster)  [unwired: 1 out]
                }
                frame "All Breaker Tick Limit" {
                  n116 = call "Command Reply.vi"("Error In"=w364, "Error?"=FALSE, "String"=w369, "Network Info"=w370) -> ("error out"=w367:errorcluster, "TCP Network Connection out"=w368:refnum<k5>)  [unwired: 6 in]
                  n117 = call-poly "TCP Read Length and Value.vi"("error in (no error)"=w367, "TCP Network Connection in"=w368) -> ("error out"=w362:errorcluster, "Output"=w365:u32)  [unwired: 7 in, 1 out]
                  n118 = xnode "Read/Write Control"("FPGA VI Reference In"=w366, "error in"=w362, "All Breaker Tick Limit"=w365) -> ("error out"=w363:errorcluster)  [unwired: 1 out]
                }
                frame "VT Quench Volt Limit" {
                  n119 = call "Command Reply.vi"("Error In"=w375, "Error?"=FALSE, "String"=w379, "Network Info"=w380) -> ("error out"=w377:errorcluster, "TCP Network Connection out"=w378:refnum<k5>)  [unwired: 6 in]
                  n120 = call-poly "TCP Read Length and Value.vi"("error in (no error)"=w377, "TCP Network Connection in"=w378) -> ("error out"=w373:errorcluster, "Output"=w372:dbl)  [unwired: 7 in, 1 out]
                  n121 = xnode "Read/Write Control"("FPGA VI Reference In"=w376, "error in"=w373, "VT Quench Volt Limit"=w372) -> ("error out"=w374:errorcluster)  [unwired: 1 out]
                }
                frame "Joint Volt Limit" {
                  n122 = call "Command Reply.vi"("Error In"=w384, "Error?"=FALSE, "String"=w389, "Network Info"=w390) -> ("error out"=w387:errorcluster, "TCP Network Connection out"=w388:refnum<k5>)  [unwired: 6 in]
                  n123 = call-poly "TCP Read Length and Value.vi"("error in (no error)"=w387, "TCP Network Connection in"=w388) -> ("error out"=w382:errorcluster, "Output"=w385:dbl)  [unwired: 7 in, 1 out]
                  n124 = xnode "Read/Write Control"("FPGA VI Reference In"=w386, "error in"=w382, "Joint Volt Limit"=w385) -> ("error out"=w383:errorcluster)  [unwired: 1 out]
                }
                frame "CoWound Volt Limit" {
                  n125 = call "Command Reply.vi"("Error In"=w395, "Error?"=FALSE, "String"=w399, "Network Info"=w400) -> ("error out"=w397:errorcluster, "TCP Network Connection out"=w398:refnum<k5>)  [unwired: 6 in]
                  n126 = call-poly "TCP Read Length and Value.vi"("error in (no error)"=w397, "TCP Network Connection in"=w398) -> ("error out"=w393:errorcluster, "Output"=w392:dbl)  [unwired: 7 in, 1 out]
                  n127 = xnode "Read/Write Control"("FPGA VI Reference In"=w396, "error in"=w393, "CoWound Volt Limit"=w392) -> ("error out"=w394:errorcluster)  [unwired: 1 out]
                }
                frame "SC Bus Limit" {
                  n128 = call "Command Reply.vi"("Error In"=w404, "Error?"=FALSE, "String"=w409, "Network Info"=w410) -> ("error out"=w407:errorcluster, "TCP Network Connection out"=w408:refnum<k5>)  [unwired: 6 in]
                  n129 = call-poly "TCP Read Length and Value.vi"("error in (no error)"=w407, "TCP Network Connection in"=w408) -> ("error out"=w402:errorcluster, "Output"=w405:dbl)  [unwired: 7 in, 1 out]
                  n130 = xnode "Read/Write Control"("FPGA VI Reference In"=w406, "error in"=w402, "SC Bus Limit"=w405) -> ("error out"=w403:errorcluster)  [unwired: 1 out]
                }
                frame "HTS Lead Trip" {
                  n131 = call "Command Reply.vi"("Error In"=w414, "Error?"=FALSE, "String"=w419, "Network Info"=w420) -> ("error out"=w417:errorcluster, "TCP Network Connection out"=w418:refnum<k5>)  [unwired: 6 in]
                  n132 = call-poly "TCP Read Length and Value.vi"("error in (no error)"=w417, "TCP Network Connection in"=w418) -> ("error out"=w412:errorcluster, "Output"=w415:dbl)  [unwired: 7 in, 1 out]
                  n133 = xnode "Read/Write Control"("FPGA VI Reference In"=w416, "error in"=w412, "HTS Lead Trip"=w415) -> ("error out"=w413:errorcluster)  [unwired: 1 out]
                }
                frame "HTS Lead FRZ" {
                  n134 = call "Command Reply.vi"("Error In"=w424, "Error?"=FALSE, "String"=w429, "Network Info"=w430) -> ("error out"=w427:errorcluster, "TCP Network Connection out"=w428:refnum<k5>)  [unwired: 6 in]
                  n135 = call-poly "TCP Read Length and Value.vi"("error in (no error)"=w427, "TCP Network Connection in"=w428) -> ("error out"=w422:errorcluster, "Output"=w425:dbl)  [unwired: 7 in, 1 out]
                  n136 = xnode "Read/Write Control"("FPGA VI Reference In"=w426, "error in"=w422, "HTS Lead FRZ"=w425) -> ("error out"=w423:errorcluster)  [unwired: 1 out]
                }
                frame "HTS Lead Warn" {
                  n137 = call "Command Reply.vi"("Error In"=w434, "Error?"=FALSE, "String"=w439, "Network Info"=w440) -> ("error out"=w437:errorcluster, "TCP Network Connection out"=w438:refnum<k5>)  [unwired: 6 in]
                  n138 = call-poly "TCP Read Length and Value.vi"("error in (no error)"=w437, "TCP Network Connection in"=w438) -> ("error out"=w432:errorcluster, "Output"=w435:dbl)  [unwired: 7 in, 1 out]
                  n139 = xnode "Read/Write Control"("FPGA VI Reference In"=w436, "error in"=w432, "HTS Lead Warn"=w435) -> ("error out"=w433:errorcluster)  [unwired: 1 out]
                }
                frame "Res Lead Limit" {
                  n140 = call "Command Reply.vi"("Error In"=w444, "Error?"=FALSE, "String"=w449, "Network Info"=w450) -> ("error out"=w447:errorcluster, "TCP Network Connection out"=w448:refnum<k5>)  [unwired: 6 in]
                  n141 = call-poly "TCP Read Length and Value.vi"("error in (no error)"=w447, "TCP Network Connection in"=w448) -> ("error out"=w442:errorcluster, "Output"=w445:dbl)  [unwired: 7 in, 1 out]
                  n142 = xnode "Read/Write Control"("FPGA VI Reference In"=w446, "error in"=w442, "Res Lead Limit"=w445) -> ("error out"=w443:errorcluster)  [unwired: 1 out]
                }
                frame "DAQ Cycle Ticks" {
                  n143 = call "Command Reply.vi"("Error In"=w453, "Error?"=FALSE, "String"=w459, "Network Info"=w460) -> ("error out"=w457:errorcluster, "TCP Network Connection out"=w458:refnum<k5>)  [unwired: 6 in]
                  n144 = call-poly "TCP Read Length and Value.vi"("error in (no error)"=w457, "TCP Network Connection in"=w458) -> ("error out"=w455:errorcluster, "Output"=w454:u32)  [unwired: 7 in, 1 out]
                  n145 = xnode "Read/Write Control"("FPGA VI Reference In"=w456, "error in"=w455, "DAQ Cycle Ticks"=w454) -> ("error out"=w452:errorcluster)  [unwired: 1 out]
                }
                frame "Res Mag dI/dt Delay" {
                  n146 = call "Command Reply.vi"("Error In"=w463, "Error?"=FALSE, "String"=w469, "Network Info"=w470) -> ("error out"=w467:errorcluster, "TCP Network Connection out"=w468:refnum<k5>)  [unwired: 6 in]
                  n147 = call-poly "TCP Read Length and Value.vi"("error in (no error)"=w467, "TCP Network Connection in"=w468) -> ("error out"=w465:errorcluster, "Output"=w464:u32)  [unwired: 7 in, 1 out]
                  n148 = xnode "Read/Write Control"("FPGA VI Reference In"=w466, "error in"=w465, "Res Mag dI/dt Delay"=w464) -> ("error out"=w462:errorcluster)  [unwired: 1 out]
                }
                frame "dI/dT Scaling" {
                  n149 = call "Command Reply.vi"("Error In"=w474, "Error?"=FALSE, "String"=w479, "Network Info"=w480) -> ("error out"=w477:errorcluster, "TCP Network Connection out"=w478:refnum<k5>)  [unwired: 6 in]
                  n150 = call-poly "TCP Read Length and Value.vi"("error in (no error)"=w477, "TCP Network Connection in"=w478) -> ("error out"=w472:errorcluster, "Output"=w475:dbl)  [unwired: 7 in, 1 out]
                  n151 = xnode "Read/Write Control"("FPGA VI Reference In"=w476, "error in"=w472, "dI/dT scaling"=w475) -> ("error out"=w473:errorcluster)  [unwired: 1 out]
                }
                frame "Pressure Inlet Limit (BarA)" {
                  n152 = call "Command Reply.vi"("Error In"=w484, "Error?"=FALSE, "String"=w489, "Network Info"=w490) -> ("error out"=w487:errorcluster, "TCP Network Connection out"=w488:refnum<k5>)  [unwired: 6 in]
                  n153 = call-poly "TCP Read Length and Value.vi"("error in (no error)"=w487, "TCP Network Connection in"=w488) -> ("error out"=w482:errorcluster, "Output"=w485:dbl)  [unwired: 7 in, 1 out]
                  n154 = xnode "Read/Write Control"("FPGA VI Reference In"=w486, "error in"=w482, "Pressure Inlet Limit (BarA)"=w485) -> ("error out"=w483:errorcluster)  [unwired: 1 out]
                }
                frame "Pressure Outlet Limit (BarA)" {
                  n155 = call "Command Reply.vi"("Error In"=w494, "Error?"=FALSE, "String"=w499, "Network Info"=w500) -> ("error out"=w497:errorcluster, "TCP Network Connection out"=w498:refnum<k5>)  [unwired: 6 in]
                  n156 = call-poly "TCP Read Length and Value.vi"("error in (no error)"=w497, "TCP Network Connection in"=w498) -> ("error out"=w492:errorcluster, "Output"=w495:dbl)  [unwired: 7 in, 1 out]
                  n157 = xnode "Read/Write Control"("FPGA VI Reference In"=w496, "error in"=w492, "Pressure Outlet Limit (BarA)"=w495) -> ("error out"=w493:errorcluster)  [unwired: 1 out]
                }
                frame "Pressure Inlest Cooldown Limit" {
                  n158 = call "Command Reply.vi"("Error In"=w504, "Error?"=FALSE, "String"=w509, "Network Info"=w510) -> ("error out"=w507:errorcluster, "TCP Network Connection out"=w508:refnum<k5>)  [unwired: 6 in]
                  n159 = call-poly "TCP Read Length and Value.vi"("error in (no error)"=w507, "TCP Network Connection in"=w508) -> ("error out"=w502:errorcluster, "Output"=w505:dbl)  [unwired: 7 in, 1 out]
                  n160 = xnode "Read/Write Control"("FPGA VI Reference In"=w506, "error in"=w502, "Pressure Inlet Cooldown Limit"=w505) -> ("error out"=w503:errorcluster)  [unwired: 1 out]
                }
                frame "Pressure Outlet Cooldown Limit" {
                  n161 = call "Command Reply.vi"("Error In"=w514, "Error?"=FALSE, "String"=w519, "Network Info"=w520) -> ("error out"=w517:errorcluster, "TCP Network Connection out"=w518:refnum<k5>)  [unwired: 6 in]
                  n162 = call-poly "TCP Read Length and Value.vi"("error in (no error)"=w517, "TCP Network Connection in"=w518) -> ("error out"=w512:errorcluster, "Output"=w515:dbl)  [unwired: 7 in, 1 out]
                  n163 = xnode "Read/Write Control"("FPGA VI Reference In"=w516, "error in"=w512, "Pressure Outlet Cooldown Limit"=w515) -> ("error out"=w513:errorcluster)  [unwired: 1 out]
                }
                frame "Bore Tube Volt Limit" {
                  n164 = call "Command Reply.vi"("Error In"=w524, "Error?"=FALSE, "String"=w529, "Network Info"=w530) -> ("error out"=w527:errorcluster, "TCP Network Connection out"=w528:refnum<k5>)  [unwired: 6 in]
                  n165 = call-poly "TCP Read Length and Value.vi"("error in (no error)"=w527, "TCP Network Connection in"=w528) -> ("error out"=w522:errorcluster, "Output"=w525:dbl)  [unwired: 7 in, 1 out]
                  n166 = xnode "Read/Write Control"("FPGA VI Reference In"=w526, "error in"=w522, "Bore Tube Volt Limit"=w525) -> ("error out"=w523:errorcluster)  [unwired: 1 out]
                }
                frame "Activation Current (kA)" {
                  n167 = call "Command Reply.vi"("Error In"=w534, "Error?"=FALSE, "String"=w539, "Network Info"=w540) -> ("error out"=w537:errorcluster, "TCP Network Connection out"=w538:refnum<k5>)  [unwired: 6 in]
                  n168 = call-poly "TCP Read Length and Value.vi"("error in (no error)"=w537, "TCP Network Connection in"=w538) -> ("error out"=w532:errorcluster, "Output"=w535:dbl)  [unwired: 7 in, 1 out]
                  n169 = xnode "Read/Write Control"("FPGA VI Reference In"=w536, "error in"=w532, "Activation Current (kA)"=w535) -> ("error out"=w533:errorcluster)  [unwired: 1 out]
                }
                frame "LN2 Filter Size" {
                  n170 = call "Command Reply.vi"("Error In"=w543, "Error?"=FALSE, "String"=w549, "Network Info"=w550) -> ("error out"=w547:errorcluster, "TCP Network Connection out"=w548:refnum<k5>)  [unwired: 6 in]
                  n171 = call-poly "TCP Read Length and Value.vi"("error in (no error)"=w547, "TCP Network Connection in"=w548) -> ("error out"=w545:errorcluster, "Output"=w544:i16)  [unwired: 7 in, 1 out]
                  n172 = xnode "Read/Write Control"("FPGA VI Reference In"=w546, "error in"=w545, "Ln2 Filter Size"=w544) -> ("error out"=w542:errorcluster)  [unwired: 1 out]
                }
                frame "# Consecutive Zeros Fault" {
                  n173 = call "Command Reply.vi"("Error In"=w553, "Error?"=FALSE, "String"=w559, "Network Info"=w560) -> ("error out"=w557:errorcluster, "TCP Network Connection out"=w558:refnum<k5>)  [unwired: 6 in]
                  n174 = call-poly "TCP Read Length and Value.vi"("error in (no error)"=w557, "TCP Network Connection in"=w558) -> ("error out"=w555:errorcluster, "Output"=w554:i16)  [unwired: 7 in, 1 out]
                  n175 = xnode "Read/Write Control"("FPGA VI Reference In"=w556, "error in"=w555, "# Consecutive Zeros Fault"=w554) -> ("error out"=w552:errorcluster)  [unwired: 1 out]
                }
                frame "Digitize Convert Ticks" {
                  n176 = call "Command Reply.vi"("Error In"=w563, "Error?"=FALSE, "String"=w569, "Network Info"=w570) -> ("error out"=w567:errorcluster, "TCP Network Connection out"=w568:refnum<k5>)  [unwired: 6 in]
                  n177 = call-poly "TCP Read Length and Value.vi"("error in (no error)"=w567, "TCP Network Connection in"=w568) -> ("error out"=w565:errorcluster, "Output"=w564:u32)  [unwired: 7 in, 1 out]
                  n178 = xnode "Read/Write Control"("FPGA VI Reference In"=w566, "error in"=w565, "Digitize Convert Ticks"=w564) -> ("error out"=w562:errorcluster)  [unwired: 1 out]
                }
                frame "Digitize Reset Ticks" {
                  n179 = call "Command Reply.vi"("Error In"=w573, "Error?"=FALSE, "String"=w579, "Network Info"=w580) -> ("error out"=w577:errorcluster, "TCP Network Connection out"=w578:refnum<k5>)  [unwired: 6 in]
                  n180 = call-poly "TCP Read Length and Value.vi"("error in (no error)"=w577, "TCP Network Connection in"=w578) -> ("error out"=w575:errorcluster, "Output"=w574:u32)  [unwired: 7 in, 1 out]
                  n181 = xnode "Read/Write Control"("FPGA VI Reference In"=w576, "error in"=w575, "Digitize Reset Ticks"=w574) -> ("error out"=w572:errorcluster)  [unwired: 1 out]
                }
                frame "Convert Clock Ticks" {
                  n182 = call "Command Reply.vi"("Error In"=w583, "Error?"=FALSE, "String"=w589, "Network Info"=w590) -> ("error out"=w587:errorcluster, "TCP Network Connection out"=w588:refnum<k5>)  [unwired: 6 in]
                  n183 = call-poly "TCP Read Length and Value.vi"("error in (no error)"=w587, "TCP Network Connection in"=w588) -> ("error out"=w585:errorcluster, "Output"=w584:u32)  [unwired: 7 in, 1 out]
                  n184 = xnode "Read/Write Control"("FPGA VI Reference In"=w586, "error in"=w585, "Convert Clock Ticks"=w584) -> ("error out"=w582:errorcluster)  [unwired: 1 out]
                }
                frame "Digitize Read Delay Ticks" {
                  n185 = call "Command Reply.vi"("Error In"=w593, "Error?"=FALSE, "String"=w599, "Network Info"=w600) -> ("error out"=w597:errorcluster, "TCP Network Connection out"=w598:refnum<k5>)  [unwired: 6 in]
                  n186 = call-poly "TCP Read Length and Value.vi"("error in (no error)"=w597, "TCP Network Connection in"=w598) -> ("error out"=w595:errorcluster, "Output"=w594:u32)  [unwired: 7 in, 1 out]
                  n187 = xnode "Read/Write Control"("FPGA VI Reference In"=w596, "error in"=w595, "Digitize Read Delay Ticks"=w594) -> ("error out"=w592:errorcluster)  [unwired: 1 out]
                }
                frame "Digitize # Bits" {
                  n188 = call "Command Reply.vi"("Error In"=w603, "Error?"=FALSE, "String"=w609, "Network Info"=w610) -> ("error out"=w607:errorcluster, "TCP Network Connection out"=w608:refnum<k5>)  [unwired: 6 in]
                  n189 = call-poly "TCP Read Length and Value.vi"("error in (no error)"=w607, "TCP Network Connection in"=w608) -> ("error out"=w605:errorcluster, "Output"=w604:u32)  [unwired: 7 in, 1 out]
                  n190 = xnode "Read/Write Control"("FPGA VI Reference In"=w606, "error in"=w605, "Digitize # Bits"=w604) -> ("error out"=w602:errorcluster)  [unwired: 1 out]
                }
                frame "Low Current (kA)" {
                  n191 = call "Command Reply.vi"("Error In"=w614, "Error?"=FALSE, "String"=w619, "Network Info"=w620) -> ("error out"=w617:errorcluster, "TCP Network Connection out"=w618:refnum<k5>)  [unwired: 6 in]
                  n192 = call-poly "TCP Read Length and Value.vi"("error in (no error)"=w617, "TCP Network Connection in"=w618) -> ("error out"=w615:errorcluster, "Output"=w612:dbl)  [unwired: 7 in, 1 out]
                  n193 = xnode "Read/Write Control"("FPGA VI Reference In"=w616, "error in"=w615, "Low Current (kA)"=w612) -> ("error out"=w613:errorcluster)  [unwired: 1 out]
                }
                frame "Magnet Configuration Data" {
                  n194 = call "Command Reply.vi"("Error In"=w629, "Error?"=FALSE, "String"=w633, "Network Info"=w634) -> ("error out"=w631:errorcluster, "TCP Network Connection out"=w632:refnum<k5>)  [unwired: 6 in]
                  n195 = call-poly "TCP Read Length and Value.vi"("error in (no error)"=w631, "TCP Network Connection in"=w632) -> ("error out"=w627:errorcluster, "Output"=w623:string)  [unwired: 7 in, 1 out]
                  n196 = Unflatten From String(type=T4 {"#Coils"=4, "Coil Inductances"=[0.10000002384185791, 0.3999999761581421, 0.6000000238418579, 1.199999988079071], "Max Coil Currents"=[19.899999976158142, 19.899999976158142, 19.899999976158142, 19.899999976158142], "Max Coil Volt Dev"=[1.800000011920929, 2.100000023841858, 3.100000023841858, 2.600000023841858], "Coil A Coefficients"=[0.8209999799728394, 0.00010001659393310547, 5.960464477539063e-08], "Coil B Coefficients"=[0.8999999761581421, 0.00019997358322143555, 2.9802322387695312e-06], "Coil C Coefficients"=[1.100000023841858, 0.0, 0.0], "Coil D Coefficients"=[1.0, 0.0009999871253967285, 0.0], "Max Coil Temp"=[100.0, 80.0, 80.0, 60.0], " Pressure Range"=[29.30000001192093, 32.30000001192093], "Temp Coef"=[0.0031999945640563965, 0.0031999945640563965, 0.0029000043869018555, 0.004100024700164795], "Offsets"=[0.0, 0.0, -5.0, -5.0, 0.0, 0.0, 0.0, 0.0, 0.0, 0.0, 0.0, 0.0, 0.0, 0.0, 0.0], "Scale Factors"=[20.0, 20.0, 4.2670000195503235, 4.269999980926514, 4.0, 1.0, 1.0, 1.0, 1.0, 1.0, -2.0, 30.08600002527237, 29.861999988555908, 35.50199997425079, 35.56999999284744]} ("Magnet Configuration Data"), binary string=w623, data includes array or string size? (T)=FALSE, error in (no error)=w627) -> (value=w625:T4, error out=w626:errorcluster)  [unwired: 1 in, 1 out]
                  n197 = xnode "Read/Write Control"("FPGA VI Reference In"=w630, "error in"=w626, "Magnet Configuration Data"=w625) -> ("error out"=w628:errorcluster)  [unwired: 1 out]
                }
                frame "Signal Injection On" {
                  n198 = call "Command Reply.vi"("Error In"=w640, "Error?"=FALSE, "String"=w643, "Network Info"=w644) -> ("error out"=w641:errorcluster, "TCP Network Connection out"=w642:refnum<k5>)  [unwired: 6 in]
                  n199 = call-poly "TCP Read Length and Value.vi"("error in (no error)"=w641, "TCP Network Connection in"=w642) -> ("error out"=w637:errorcluster, "Output"=w638:bool)  [unwired: 7 in, 1 out]
                  n200 = xnode "Read/Write Control"("FPGA VI Reference In"=w639, "error in"=w637, "Signal Injection On"=w638) -> ("error out"=w636:errorcluster)  [unwired: 1 out]
                }
                frame "Inject Frequency (Hz)" {
                  n201 = call "Command Reply.vi"("Error In"=w649, "Error?"=FALSE, "String"=w653, "Network Info"=w654) -> ("error out"=w651:errorcluster, "TCP Network Connection out"=w652:refnum<k5>)  [unwired: 6 in]
                  n202 = call-poly "TCP Read Length and Value.vi"("error in (no error)"=w651, "TCP Network Connection in"=w652) -> ("error out"=w647:errorcluster, "Output"=w646:dbl)  [unwired: 7 in, 1 out]
                  n203 = xnode "Read/Write Control"("FPGA VI Reference In"=w650, "error in"=w647, "Inject frequency (Hz)"=w646) -> ("error out"=w648:errorcluster)  [unwired: 1 out]
                }
                frame "Inject Offset" {
                  n204 = call "Command Reply.vi"("Error In"=w659, "Error?"=FALSE, "String"=w663, "Network Info"=w664) -> ("error out"=w661:errorcluster, "TCP Network Connection out"=w662:refnum<k5>)  [unwired: 6 in]
                  n205 = call-poly "TCP Read Length and Value.vi"("error in (no error)"=w661, "TCP Network Connection in"=w662) -> ("error out"=w657:errorcluster, "Output"=w656:dbl)  [unwired: 7 in, 1 out]
                  n206 = xnode "Read/Write Control"("FPGA VI Reference In"=w660, "error in"=w657, "Inject Offset"=w656) -> ("error out"=w658:errorcluster)  [unwired: 1 out]
                }
                frame "Inject Channel" {
                  n207 = call "Command Reply.vi"("Error In"=w669, "Error?"=FALSE, "String"=w673, "Network Info"=w674) -> ("error out"=w671:errorcluster, "TCP Network Connection out"=w672:refnum<k5>)  [unwired: 6 in]
                  n208 = call-poly "TCP Read Length and Value.vi"("error in (no error)"=w671, "TCP Network Connection in"=w672) -> ("error out"=w667:errorcluster, "Output"=w666:i32)  [unwired: 7 in, 1 out]
                  n209 = xnode "Read/Write Control"("FPGA VI Reference In"=w670, "error in"=w667, "Inject Channel"=w666) -> ("error out"=w668:errorcluster)  [unwired: 1 out]
                }
                frame "Low Current Ticks" {
                  n210 = call "Command Reply.vi"("Error In"=w679, "Error?"=FALSE, "String"=w683, "Network Info"=w684) -> ("error out"=w681:errorcluster, "TCP Network Connection out"=w682:refnum<k5>)  [unwired: 6 in]
                  n211 = call-poly "TCP Read Length and Value.vi"("error in (no error)"=w681, "TCP Network Connection in"=w682) -> ("error out"=w677:errorcluster, "Output"=w676:u32)  [unwired: 7 in, 1 out]
                  n212 = xnode "Read/Write Control"("FPGA VI Reference In"=w680, "error in"=w677, "Low Current Ticks"=w676) -> ("error out"=w678:errorcluster)  [unwired: 1 out]
                }
                frame "Ticks to Close Relief" {
                  n213 = call "Command Reply.vi"("Error In"=w689, "Error?"=FALSE, "String"=w693, "Network Info"=w694) -> ("error out"=w691:errorcluster, "TCP Network Connection out"=w692:refnum<k5>)  [unwired: 6 in]
                  n214 = call-poly "TCP Read Length and Value.vi"("error in (no error)"=w691, "TCP Network Connection in"=w692) -> ("error out"=w687:errorcluster, "Output"=w686:u32)  [unwired: 7 in, 1 out]
                  n215 = xnode "Read/Write Control"("FPGA VI Reference In"=w690, "error in"=w687, "Ticks to Close Relief"=w686) -> ("error out"=w688:errorcluster)  [unwired: 1 out]
                }
                frame "Delay Ticks Between Bkr Reset" {
                  n216 = call "Command Reply.vi"("Error In"=w699, "Error?"=FALSE, "String"=w703, "Network Info"=w704) -> ("error out"=w701:errorcluster, "TCP Network Connection out"=w702:refnum<k5>)  [unwired: 6 in]
                  n217 = call-poly "TCP Read Length and Value.vi"("error in (no error)"=w701, "TCP Network Connection in"=w702) -> ("error out"=w697:errorcluster, "Output"=w696:u32)  [unwired: 7 in, 1 out]
                  n218 = xnode "Read/Write Control"("FPGA VI Reference In"=w700, "error in"=w697, "Delay Ticks Between Bkr Reset"=w696) -> ("error out"=w698:errorcluster)  [unwired: 1 out]
                }
                frame "Breaker Reset Ticks" {
                  n219 = call "Command Reply.vi"("Error In"=w709, "Error?"=FALSE, "String"=w713, "Network Info"=w714) -> ("error out"=w711:errorcluster, "TCP Network Connection out"=w712:refnum<k5>)  [unwired: 6 in]
                  n220 = call-poly "TCP Read Length and Value.vi"("error in (no error)"=w711, "TCP Network Connection in"=w712) -> ("error out"=w707:errorcluster, "Output"=w706:u32)  [unwired: 7 in, 1 out]
                  n221 = xnode "Read/Write Control"("FPGA VI Reference In"=w710, "error in"=w707, "Breaker Reset Ticks"=w706) -> ("error out"=w708:errorcluster)  [unwired: 1 out]
                }
                frame "PS Enable Reset Ticks" {
                  n222 = call "Command Reply.vi"("Error In"=w719, "Error?"=FALSE, "String"=w723, "Network Info"=w724) -> ("error out"=w721:errorcluster, "TCP Network Connection out"=w722:refnum<k5>)  [unwired: 6 in]
                  n223 = call-poly "TCP Read Length and Value.vi"("error in (no error)"=w721, "TCP Network Connection in"=w722) -> ("error out"=w717:errorcluster, "Output"=w716:u32)  [unwired: 7 in, 1 out]
                  n224 = xnode "Read/Write Control"("FPGA VI Reference In"=w720, "error in"=w717, "PS Enable Reset Ticks"=w716) -> ("error out"=w718:errorcluster)  [unwired: 1 out]
                }
                frame "Reset Digitizer Ticks" {
                  n225 = call "Command Reply.vi"("Error In"=w729, "Error?"=FALSE, "String"=w733, "Network Info"=w734) -> ("error out"=w731:errorcluster, "TCP Network Connection out"=w732:refnum<k5>)  [unwired: 6 in]
                  n226 = call-poly "TCP Read Length and Value.vi"("error in (no error)"=w731, "TCP Network Connection in"=w732) -> ("error out"=w727:errorcluster, "Output"=w726:u32)  [unwired: 7 in, 1 out]
                  n227 = xnode "Read/Write Control"("FPGA VI Reference In"=w730, "error in"=w727, "Reset Digitizer Ticks"=w726) -> ("error out"=w728:errorcluster)  [unwired: 1 out]
                }
                frame "Low Current Delay Factor" {
                  n228 = call "Command Reply.vi"("Error In"=w739, "Error?"=FALSE, "String"=w743, "Network Info"=w744) -> ("error out"=w741:errorcluster, "TCP Network Connection out"=w742:refnum<k5>)  [unwired: 6 in]
                  n229 = call-poly "TCP Read Length and Value.vi"("error in (no error)"=w741, "TCP Network Connection in"=w742) -> ("error out"=w737:errorcluster, "Output"=w736:u16)  [unwired: 7 in, 1 out]
                  n230 = xnode "Read/Write Control"("FPGA VI Reference In"=w740, "error in"=w737, "Low Current Delay Factor"=w736) -> ("error out"=w738:errorcluster)  [unwired: 1 out]
                }
                frame "Reset Digitizers" {
                  n231 = call "Command Reply.vi"("Error In"=w752, "Error?"=FALSE, "String"=w755, "Network Info"=w756) -> ("error out"=w753:errorcluster, "TCP Network Connection out"=w754:refnum<k5>)  [unwired: 6 in]
                  n232 = call-poly "TCP Read Length and Value.vi"("error in (no error)"=w753, "TCP Network Connection in"=w754) -> ("error out"=w747:errorcluster, "Output"=w750:bool)  [unwired: 7 in, 1 out]
                  n233 = xnode "Read/Write Control"("FPGA VI Reference In"=w749, "error in"=w747, "Reset Digitizers"=w750) -> ("FPGA VI Reference Out"=w748:T3, "error out"=w746:errorcluster)
                  n234 = call "Stop and Empty FIFOs.vi"("error in"=w746, "Refnum in"=w748) -> ("error out"=w751:errorcluster)  [unwired: 8 in, 1 out]
                }
                frame "Reset PS Enable" {
                  n235 = call "Command Reply.vi"("Error In"=w762, "Error?"=FALSE, "String"=w765, "Network Info"=w766) -> ("error out"=w763:errorcluster, "TCP Network Connection out"=w764:refnum<k5>)  [unwired: 6 in]
                  n236 = call-poly "TCP Read Length and Value.vi"("error in (no error)"=w763, "TCP Network Connection in"=w764) -> ("error out"=w759:errorcluster, "Output"=w761:bool)  [unwired: 7 in, 1 out]
                  n237 = xnode "Read/Write Control"("FPGA VI Reference In"=w760, "error in"=w759, "Reset PS Enable"=w761) -> ("error out"=w758:errorcluster)  [unwired: 1 out]
                }
                frame "Reset Breaker" {
                  n238 = call "Command Reply.vi"("Error In"=w772, "Error?"=FALSE, "String"=w775, "Network Info"=w776) -> ("error out"=w773:errorcluster, "TCP Network Connection out"=w774:refnum<k5>)  [unwired: 6 in]
                  n239 = call-poly "TCP Read Length and Value.vi"("error in (no error)"=w773, "TCP Network Connection in"=w774) -> ("error out"=w769:errorcluster, "Output"=w771:bool)  [unwired: 7 in, 1 out]
                  n240 = xnode "Read/Write Control"("FPGA VI Reference In"=w770, "error in"=w769, "Reset Breaker"=w771) -> ("error out"=w768:errorcluster)  [unwired: 1 out]
                }
                frame "Cooldown Mode" {
                  n241 = call "Command Reply.vi"("Error In"=w782, "Error?"=FALSE, "String"=w785, "Network Info"=w786) -> ("error out"=w783:errorcluster, "TCP Network Connection out"=w784:refnum<k5>)  [unwired: 6 in]
                  n242 = call-poly "TCP Read Length and Value.vi"("error in (no error)"=w783, "TCP Network Connection in"=w784) -> ("error out"=w779:errorcluster, "Output"=w781:bool)  [unwired: 7 in, 1 out]
                  n243 = xnode "Read/Write Control"("FPGA VI Reference In"=w780, "error in"=w779, "Cooldown Mode"=w781) -> ("error out"=w778:errorcluster)  [unwired: 1 out]
                }
                frame "Calibrate" {
                  n244 = call "Command Reply.vi"("Error In"=w790, "Error?"=FALSE, "String"=w795, "Network Info"=w796) -> ("error out"=w793:errorcluster, "TCP Network Connection out"=w794:refnum<k5>)  [unwired: 6 in]
                  n245 = call-poly "TCP Read Length and Value.vi"("error in (no error)"=w793, "TCP Network Connection in"=w794) -> ("error out"=w788:errorcluster, "Output"=w791:bool)  [unwired: 7 in, 1 out]
                  n246 = case shown="True" w791 {
                    tunnel: w792 -> [_ w803]
                    tunnel: w788 -> [w798 w802]
                    tunnel: [w798 w801] -> w789
                    frame False {
                    }
                    frame True {
                      n247 = Get Date/Time In Seconds() -> (seconds since 1Jan1904=w799:timestamp)
                      n248 = global write "RT Host Globals.vi" "Calibration DateStamp"(w799) -> ()
                      n249 = xnode "Read/Write Control"("FPGA VI Reference In"=w803, "error in"=w802, "Input Select"=T6."Zero Voltage") -> ("error out"=w801:errorcluster)  [unwired: 1 out]
                    }
                  }
                }
                frame "Notification Email" {
                  n250 = call "Command Reply.vi"("Error In"=w806, "Error?"=FALSE, "String"=w809, "Network Info"=w810) -> ("error out"=w807:errorcluster, "TCP Network Connection out"=w808:refnum<k5>)  [unwired: 6 in]
                  n251 = call-poly "TCP Read Length and Value.vi"("error in (no error)"=w807, "TCP Network Connection in"=w808) -> ("error out"=w805:errorcluster, "Output"=w804:string)  [unwired: 7 in, 1 out]
                  n252 = global write "RT Host Globals.vi" "Notification Email"(w804) -> ()
                }
              }
            }
          }
        }
        frame "GET" {
          n253 = case shown="\"Notification Email\"" w814 {
            tunnel: w812 -> [w821 w831 w842 w853 w864 w875 w886 w897 w908 w919 w930 w940 w950 w960 w970 w980 w990 w1000 w1011 w1022 w1033 w1044 w1055 w1066 w1077 w1088 w1098 w1108 w1119 w1129 w1140 w1151 w1162 w1173 w1184 w1195 w1205 w1215 w1225 w1235 w1245 w1255 w1265 w1277 w1288 w1298 w1309 w1319 w1329 w1339 w1350 w1360 w1370 w1380 w1390 w1400 w1410 w1420 w1429 w1439 w1454 w1467 w1475 w1483 w1491]
            tunnel: w817 -> [_ w833 w844 w855 w866 w877 w888 w899 w910 w921 w932 w942 w952 w962 w972 w982 w992 w1002 w1013 w1024 w1035 w1046 w1057 w1068 w1079 w1090 w1100 w1110 w1121 w1131 w1142 w1153 w1164 w1175 w1186 w1197 w1207 w1217 w1227 w1237 w1247 w1257 w1267 w1279 w1283 w1300 w1311 w1321 w1331 w1341 w1352 w1362 w1372 w1382 w1392 w1402 w1412 w1422 _ _ w1449 _ _ _ _]
            tunnel: w816 -> [w820 w827 w837 w848 w859 w870 w881 w892 w903 w914 w925 w936 w946 w956 w966 w976 w986 w996 w1007 w1018 w1028 w1039 w1050 w1061 w1072 w1083 w1094 w1104 w1114 w1125 w1135 w1146 w1157 w1168 w1179 w1190 w1201 w1211 w1221 w1231 w1241 w1251 w1261 w1274 w1285 w1293 w1304 w1315 w1325 w1335 w1346 w1356 w1366 w1376 w1386 w1396 w1406 w1416 w1426 w1436 w1451 w1464 w1472 w1480 w1488]
            tunnel: w813 -> [w819 w830 w841 w852 w863 w874 w885 w896 w907 w918 w929 w939 w949 w959 w969 w979 w989 w999 w1010 w1021 w1032 w1043 w1054 w1065 w1076 w1087 w1097 w1107 w1118 w1128 w1139 w1150 w1161 w1172 w1183 w1194 w1204 w1214 w1224 w1234 w1244 w1254 w1264 w1276 w1287 w1297 w1308 w1318 w1328 w1338 w1349 w1359 w1369 w1379 w1389 w1399 w1409 w1419 w1428 w1438 w1453 w1466 w1474 w1482 w1490]
            tunnel: [w818 w824 w834 w847 w858 w869 w880 w891 w902 w913 w924 w935 w945 w955 w965 w975 w985 w995 w1006 w1017 w1027 w1038 w1049 w1060 w1071 w1082 w1093 w1103 w1113 w1124 w1134 w1145 w1156 w1167 w1178 w1189 w1200 w1210 w1220 w1230 w1240 w1250 w1260 w1273 w1284 w1292 w1303 w1314 w1324 w1334 w1345 w1355 w1365 w1375 w1385 w1395 w1405 w1415 w1425 w1435 w1450 w1463 w1471 w1479 w1487] -> w815
            frame Default {
              n254 = call "Command Reply.vi"("Error In"=w820, "Error?"=TRUE, "String"=w819, "Network Info"=w821) -> ("error out"=w818:errorcluster)  [unwired: 6 in, 1 out]
            }
            frame "Layer Scale Factors" {
              n255 = call "Command Reply.vi"("Error In"=w827, "Error?"=FALSE, "String"=w830, "Network Info"=w831) -> ("error out"=w826:errorcluster, "TCP Network Connection out"=w828:refnum<k5>)  [unwired: 6 in]
              n256 = xnode "Read/Write Control"("FPGA VI Reference In"=w833, "error in"=w826) -> ("error out"=w825:errorcluster, "Layer Scale Factors"=w829:fxp<+/-,38,12>[])  [unwired: 1 out]
              n257 = To Double Precision Float(number=w829) -> (double precision float=w823:dbl[])
              n258 = call-poly "TCP Write Length and Data.vi"("Error In"=w825, "Data"=w823, "connection ID"=w828) -> ("Error Out"=w824:errorcluster)  [unwired: 7 in, 1 out]
            }
            frame "Fudge Factors" {
              n259 = call "Command Reply.vi"("Error In"=w837, "Error?"=FALSE, "String"=w841, "Network Info"=w842) -> ("error out"=w836:errorcluster, "TCP Network Connection out"=w838:refnum<k5>)  [unwired: 6 in]
              n260 = xnode "Read/Write Control"("FPGA VI Reference In"=w844, "error in"=w836) -> ("error out"=w835:errorcluster, "Fudge Factors"=w839:fxp<+/-,32,3>[])  [unwired: 1 out]
              n261 = To Double Precision Float(number=w839) -> (double precision float=w840:dbl[])
              n262 = call-poly "TCP Write Length and Data.vi"("Error In"=w835, "Data"=w840, "connection ID"=w838) -> ("Error Out"=w834:errorcluster)  [unwired: 7 in, 1 out]
            }
            frame "Co-Wound Scale Factor" {
              n263 = call "Command Reply.vi"("Error In"=w848, "Error?"=FALSE, "String"=w852, "Network Info"=w853) -> ("error out"=w845:errorcluster, "TCP Network Connection out"=w849:refnum<k5>)  [unwired: 6 in]
              n264 = xnode "Read/Write Control"("FPGA VI Reference In"=w855, "error in"=w845) -> ("error out"=w846:errorcluster, "Co-Wound Scale Factor"=w850:fxp<+/-,38,12>)  [unwired: 1 out]
              n265 = To Double Precision Float(number=w850) -> (double precision float=w851:dbl)
              n266 = call-poly "TCP Write Length and Data.vi"("Error In"=w846, "Data"=w851, "connection ID"=w849) -> ("Error Out"=w847:errorcluster)  [unwired: 7 in, 1 out]
            }
            frame "Co-Wound Asymmetry Factor" {
              n267 = call "Command Reply.vi"("Error In"=w859, "Error?"=FALSE, "String"=w863, "Network Info"=w864) -> ("error out"=w856:errorcluster, "TCP Network Connection out"=w860:refnum<k5>)  [unwired: 6 in]
              n268 = xnode "Read/Write Control"("FPGA VI Reference In"=w866, "error in"=w856) -> ("error out"=w857:errorcluster, "Co-Wound Asymmetry Factor"=w861:fxp<+/-,16,0>)  [unwired: 1 out]
              n269 = To Double Precision Float(number=w861) -> (double precision float=w862:dbl)
              n270 = call-poly "TCP Write Length and Data.vi"("Error In"=w857, "Data"=w862, "connection ID"=w860) -> ("Error Out"=w858:errorcluster)  [unwired: 7 in, 1 out]
            }
            frame "Dump Resistor Scale Factor" {
              n271 = call "Command Reply.vi"("Error In"=w870, "Error?"=FALSE, "String"=w874, "Network Info"=w875) -> ("error out"=w867:errorcluster, "TCP Network Connection out"=w871:refnum<k5>)  [unwired: 6 in]
              n272 = xnode "Read/Write Control"("FPGA VI Reference In"=w877, "error in"=w867) -> ("error out"=w868:errorcluster, "Dump Resistor Scale Factor"=w872:fxp<+/-,38,12>)  [unwired: 1 out]
              n273 = To Double Precision Float(number=w872) -> (double precision float=w873:dbl)
              n274 = call-poly "TCP Write Length and Data.vi"("Error In"=w868, "Data"=w873, "connection ID"=w871) -> ("Error Out"=w869:errorcluster)  [unwired: 7 in, 1 out]
            }
            frame "Joint Scale Factors" {
              n275 = call "Command Reply.vi"("Error In"=w881, "Error?"=FALSE, "String"=w885, "Network Info"=w886) -> ("error out"=w878:errorcluster, "TCP Network Connection out"=w882:refnum<k5>)  [unwired: 6 in]
              n276 = xnode "Read/Write Control"("FPGA VI Reference In"=w888, "error in"=w878) -> ("error out"=w879:errorcluster, "Joint Scale Factors"=w883:fxp<+/-,38,12>[])  [unwired: 1 out]
              n277 = To Double Precision Float(number=w883) -> (double precision float=w884:dbl[])
              n278 = call-poly "TCP Write Length and Data.vi"("Error In"=w879, "Data"=w884, "connection ID"=w882) -> ("Error Out"=w880:errorcluster)  [unwired: 7 in, 1 out]
            }
            frame "SC Bus Scale" {
              n279 = call "Command Reply.vi"("Error In"=w892, "Error?"=FALSE, "String"=w896, "Network Info"=w897) -> ("error out"=w889:errorcluster, "TCP Network Connection out"=w893:refnum<k5>)  [unwired: 6 in]
              n280 = xnode "Read/Write Control"("FPGA VI Reference In"=w899, "error in"=w889) -> ("error out"=w890:errorcluster, "SC Bus Scale"=w894:fxp<+/-,38,12>[])  [unwired: 1 out]
              n281 = To Double Precision Float(number=w894) -> (double precision float=w895:dbl[])
              n282 = call-poly "TCP Write Length and Data.vi"("Error In"=w890, "Data"=w895, "connection ID"=w893) -> ("Error Out"=w891:errorcluster)  [unwired: 7 in, 1 out]
            }
            frame "HTS Resistance (nOhm)" {
              n283 = call "Command Reply.vi"("Error In"=w903, "Error?"=FALSE, "String"=w907, "Network Info"=w908) -> ("error out"=w900:errorcluster, "TCP Network Connection out"=w904:refnum<k5>)  [unwired: 6 in]
              n284 = xnode "Read/Write Control"("FPGA VI Reference In"=w910, "error in"=w900) -> ("error out"=w901:errorcluster, "HTS Resistance (nOhm)"=w905:fxp<+/-,38,12>[])  [unwired: 1 out]
              n285 = To Double Precision Float(number=w905) -> (double precision float=w906:dbl[])
              n286 = call-poly "TCP Write Length and Data.vi"("Error In"=w901, "Data"=w906, "connection ID"=w904) -> ("Error Out"=w902:errorcluster)  [unwired: 7 in, 1 out]
            }
            frame "HTS Offset (microV)" {
              n287 = call "Command Reply.vi"("Error In"=w914, "Error?"=FALSE, "String"=w918, "Network Info"=w919) -> ("error out"=w911:errorcluster, "TCP Network Connection out"=w915:refnum<k5>)  [unwired: 6 in]
              n288 = xnode "Read/Write Control"("FPGA VI Reference In"=w921, "error in"=w911) -> ("error out"=w912:errorcluster, "HTS Offset (microV)"=w916:fxp<+/-,38,12>[])  [unwired: 1 out]
              n289 = To Double Precision Float(number=w916) -> (double precision float=w917:dbl[])
              n290 = call-poly "TCP Write Length and Data.vi"("Error In"=w912, "Data"=w917, "connection ID"=w915) -> ("Error Out"=w913:errorcluster)  [unwired: 7 in, 1 out]
            }
            frame "Pressure Scale Factor" {
              n291 = call "Command Reply.vi"("Error In"=w925, "Error?"=FALSE, "String"=w929, "Network Info"=w930) -> ("error out"=w922:errorcluster, "TCP Network Connection out"=w926:refnum<k5>)  [unwired: 6 in]
              n292 = xnode "Read/Write Control"("FPGA VI Reference In"=w932, "error in"=w922) -> ("error out"=w923:errorcluster, "Pressure Scale Factor"=w927:fxp<+/-,38,12>[])  [unwired: 1 out]
              n293 = To Double Precision Float(number=w927) -> (double precision float=w928:dbl[])
              n294 = call-poly "TCP Write Length and Data.vi"("Error In"=w923, "Data"=w928, "connection ID"=w926) -> ("Error Out"=w924:errorcluster)  [unwired: 7 in, 1 out]
            }
            frame "VT Quench Tick Limit" {
              n295 = call "Command Reply.vi"("Error In"=w936, "Error?"=FALSE, "String"=w939, "Network Info"=w940) -> ("error out"=w933:errorcluster, "TCP Network Connection out"=w937:refnum<k5>)  [unwired: 6 in]
              n296 = xnode "Read/Write Control"("FPGA VI Reference In"=w942, "error in"=w933) -> ("error out"=w934:errorcluster, "VT Quench Tick Limit"=w938:u32)  [unwired: 1 out]
              n297 = call-poly "TCP Write Length and Data.vi"("Error In"=w934, "Data"=w938, "connection ID"=w937) -> ("Error Out"=w935:errorcluster)  [unwired: 7 in, 1 out]
            }
            frame "Joint Tick Limit" {
              n298 = call "Command Reply.vi"("Error In"=w946, "Error?"=FALSE, "String"=w949, "Network Info"=w950) -> ("error out"=w943:errorcluster, "TCP Network Connection out"=w947:refnum<k5>)  [unwired: 6 in]
              n299 = xnode "Read/Write Control"("FPGA VI Reference In"=w952, "error in"=w943) -> ("error out"=w944:errorcluster, "Joint Tick Limit"=w948:u32)  [unwired: 1 out]
              n300 = call-poly "TCP Write Length and Data.vi"("Error In"=w944, "Data"=w948, "connection ID"=w947) -> ("Error Out"=w945:errorcluster)  [unwired: 7 in, 1 out]
            }
            frame "CoWound Tick Limit" {
              n301 = call "Command Reply.vi"("Error In"=w956, "Error?"=FALSE, "String"=w959, "Network Info"=w960) -> ("error out"=w953:errorcluster, "TCP Network Connection out"=w957:refnum<k5>)  [unwired: 6 in]
              n302 = xnode "Read/Write Control"("FPGA VI Reference In"=w962, "error in"=w953) -> ("error out"=w954:errorcluster, "CoWound Tick Limit"=w958:u32)  [unwired: 1 out]
              n303 = call-poly "TCP Write Length and Data.vi"("Error In"=w954, "Data"=w958, "connection ID"=w957) -> ("Error Out"=w955:errorcluster)  [unwired: 7 in, 1 out]
            }
            frame "SC Bus Tick Limit" {
              n304 = call "Command Reply.vi"("Error In"=w966, "Error?"=FALSE, "String"=w969, "Network Info"=w970) -> ("error out"=w963:errorcluster, "TCP Network Connection out"=w967:refnum<k5>)  [unwired: 6 in]
              n305 = xnode "Read/Write Control"("FPGA VI Reference In"=w972, "error in"=w963) -> ("error out"=w964:errorcluster, "SC Bus Tick Limit"=w968:u32)  [unwired: 1 out]
              n306 = call-poly "TCP Write Length and Data.vi"("Error In"=w964, "Data"=w968, "connection ID"=w967) -> ("Error Out"=w965:errorcluster)  [unwired: 7 in, 1 out]
            }
            frame "HTS Lead Tick Limit" {
              n307 = call "Command Reply.vi"("Error In"=w976, "Error?"=FALSE, "String"=w979, "Network Info"=w980) -> ("error out"=w973:errorcluster, "TCP Network Connection out"=w977:refnum<k5>)  [unwired: 6 in]
              n308 = xnode "Read/Write Control"("FPGA VI Reference In"=w982, "error in"=w973) -> ("error out"=w974:errorcluster, "HTS Lead Tick Limit"=w978:u32)  [unwired: 1 out]
              n309 = call-poly "TCP Write Length and Data.vi"("Error In"=w974, "Data"=w978, "connection ID"=w977) -> ("Error Out"=w975:errorcluster)  [unwired: 7 in, 1 out]
            }
            frame "Res Lead Tick Limit" {
              n310 = call "Command Reply.vi"("Error In"=w986, "Error?"=FALSE, "String"=w989, "Network Info"=w990) -> ("error out"=w983:errorcluster, "TCP Network Connection out"=w987:refnum<k5>)  [unwired: 6 in]
              n311 = xnode "Read/Write Control"("FPGA VI Reference In"=w992, "error in"=w983) -> ("error out"=w984:errorcluster, "Res Lead Tick Limit"=w988:u32)  [unwired: 1 out]
              n312 = call-poly "TCP Write Length and Data.vi"("Error In"=w984, "Data"=w988, "connection ID"=w987) -> ("Error Out"=w985:errorcluster)  [unwired: 7 in, 1 out]
            }
            frame "ResMag Tick Limit" {
              n313 = call "Command Reply.vi"("Error In"=w996, "Error?"=FALSE, "String"=w999, "Network Info"=w1000) -> ("error out"=w993:errorcluster, "TCP Network Connection out"=w997:refnum<k5>)  [unwired: 6 in]
              n314 = xnode "Read/Write Control"("FPGA VI Reference In"=w1002, "error in"=w993) -> ("error out"=w994:errorcluster, "ResMag Tick Limit"=w998:u32)  [unwired: 1 out]
              n315 = call-poly "TCP Write Length and Data.vi"("Error In"=w994, "Data"=w998, "connection ID"=w997) -> ("Error Out"=w995:errorcluster)  [unwired: 7 in, 1 out]
            }
            frame "VT Quench Volt Limit" {
              n316 = call "Command Reply.vi"("Error In"=w1007, "Error?"=FALSE, "String"=w1010, "Network Info"=w1011) -> ("error out"=w1004:errorcluster, "TCP Network Connection out"=w1008:refnum<k5>)  [unwired: 6 in]
              n317 = xnode "Read/Write Control"("FPGA VI Reference In"=w1013, "error in"=w1004) -> ("error out"=w1005:errorcluster, "VT Quench Volt Limit"=w1009:fxp<+/-,38,12>)  [unwired: 1 out]
              n318 = To Double Precision Float(number=w1009) -> (double precision float=w1003:dbl)
              n319 = call-poly "TCP Write Length and Data.vi"("Error In"=w1005, "Data"=w1003, "connection ID"=w1008) -> ("Error Out"=w1006:errorcluster)  [unwired: 7 in, 1 out]
            }
            frame "Joint Volt Limit" {
              n320 = call "Command Reply.vi"("Error In"=w1018, "Error?"=FALSE, "String"=w1021, "Network Info"=w1022) -> ("error out"=w1015:errorcluster, "TCP Network Connection out"=w1019:refnum<k5>)  [unwired: 6 in]
              n321 = xnode "Read/Write Control"("FPGA VI Reference In"=w1024, "error in"=w1015) -> ("error out"=w1016:errorcluster, "Joint Volt Limit"=w1020:fxp<+/-,38,12>)  [unwired: 1 out]
              n322 = To Double Precision Float(number=w1020) -> (double precision float=w1014:dbl)
              n323 = call-poly "TCP Write Length and Data.vi"("Error In"=w1016, "Data"=w1014, "connection ID"=w1019) -> ("Error Out"=w1017:errorcluster)  [unwired: 7 in, 1 out]
            }
            frame "CoWound Volt Limit" {
              n324 = call "Command Reply.vi"("Error In"=w1028, "Error?"=FALSE, "String"=w1032, "Network Info"=w1033) -> ("error out"=w1025:errorcluster, "TCP Network Connection out"=w1029:refnum<k5>)  [unwired: 6 in]
              n325 = xnode "Read/Write Control"("FPGA VI Reference In"=w1035, "error in"=w1025) -> ("error out"=w1026:errorcluster, "CoWound Volt Limit"=w1030:fxp<+/-,16,1>)  [unwired: 1 out]
              n326 = To Double Precision Float(number=w1030) -> (double precision float=w1031:dbl)
              n327 = call-poly "TCP Write Length and Data.vi"("Error In"=w1026, "Data"=w1031, "connection ID"=w1029) -> ("Error Out"=w1027:errorcluster)  [unwired: 7 in, 1 out]
            }
            frame "SC Bus Limit" {
              n328 = call "Command Reply.vi"("Error In"=w1039, "Error?"=FALSE, "String"=w1043, "Network Info"=w1044) -> ("error out"=w1036:errorcluster, "TCP Network Connection out"=w1040:refnum<k5>)  [unwired: 6 in]
              n329 = xnode "Read/Write Control"("FPGA VI Reference In"=w1046, "error in"=w1036) -> ("error out"=w1037:errorcluster, "SC Bus Limit"=w1041:fxp<+/-,38,12>)  [unwired: 1 out]
              n330 = To Double Precision Float(number=w1041) -> (double precision float=w1042:dbl)
              n331 = call-poly "TCP Write Length and Data.vi"("Error In"=w1037, "Data"=w1042, "connection ID"=w1040) -> ("Error Out"=w1038:errorcluster)  [unwired: 7 in, 1 out]
            }
            frame "HTS Lead Trip" {
              n332 = call "Command Reply.vi"("Error In"=w1050, "Error?"=FALSE, "String"=w1054, "Network Info"=w1055) -> ("error out"=w1047:errorcluster, "TCP Network Connection out"=w1051:refnum<k5>)  [unwired: 6 in]
              n333 = xnode "Read/Write Control"("FPGA VI Reference In"=w1057, "error in"=w1047) -> ("error out"=w1048:errorcluster, "HTS Lead Trip"=w1052:fxp<+/-,38,12>)  [unwired: 1 out]
              n334 = To Double Precision Float(number=w1052) -> (double precision float=w1053:dbl)
              n335 = call-poly "TCP Write Length and Data.vi"("Error In"=w1048, "Data"=w1053, "connection ID"=w1051) -> ("Error Out"=w1049:errorcluster)  [unwired: 7 in, 1 out]
            }
            frame "HTS Lead FRZ" {
              n336 = call "Command Reply.vi"("Error In"=w1061, "Error?"=FALSE, "String"=w1065, "Network Info"=w1066) -> ("error out"=w1058:errorcluster, "TCP Network Connection out"=w1062:refnum<k5>)  [unwired: 6 in]
              n337 = xnode "Read/Write Control"("FPGA VI Reference In"=w1068, "error in"=w1058) -> ("error out"=w1059:errorcluster, "HTS Lead FRZ"=w1063:fxp<+/-,38,12>)  [unwired: 1 out]
              n338 = To Double Precision Float(number=w1063) -> (double precision float=w1064:dbl)
              n339 = call-poly "TCP Write Length and Data.vi"("Error In"=w1059, "Data"=w1064, "connection ID"=w1062) -> ("Error Out"=w1060:errorcluster)  [unwired: 7 in, 1 out]
            }
            frame "HTS Lead Warn" {
              n340 = call "Command Reply.vi"("Error In"=w1072, "Error?"=FALSE, "String"=w1076, "Network Info"=w1077) -> ("error out"=w1069:errorcluster, "TCP Network Connection out"=w1073:refnum<k5>)  [unwired: 6 in]
              n341 = xnode "Read/Write Control"("FPGA VI Reference In"=w1079, "error in"=w1069) -> ("error out"=w1070:errorcluster, "HTS Lead Warn"=w1074:fxp<+/-,38,12>)  [unwired: 1 out]
              n342 = To Double Precision Float(number=w1074) -> (double precision float=w1075:dbl)
              n343 = call-poly "TCP Write Length and Data.vi"("Error In"=w1070, "Data"=w1075, "connection ID"=w1073) -> ("Error Out"=w1071:errorcluster)  [unwired: 7 in, 1 out]
            }
            frame "Res Lead Limit" {
              n344 = call "Command Reply.vi"("Error In"=w1083, "Error?"=FALSE, "String"=w1087, "Network Info"=w1088) -> ("error out"=w1080:errorcluster, "TCP Network Connection out"=w1084:refnum<k5>)  [unwired: 6 in]
              n345 = xnode "Read/Write Control"("FPGA VI Reference In"=w1090, "error in"=w1080) -> ("error out"=w1081:errorcluster, "Res Lead Limit"=w1085:fxp<+/-,38,12>)  [unwired: 1 out]
              n346 = To Double Precision Float(number=w1085) -> (double precision float=w1086:dbl)
              n347 = call-poly "TCP Write Length and Data.vi"("Error In"=w1081, "Data"=w1086, "connection ID"=w1084) -> ("Error Out"=w1082:errorcluster)  [unwired: 7 in, 1 out]
            }
            frame "DAQ Cycle Ticks" {
              n348 = call "Command Reply.vi"("Error In"=w1094, "Error?"=FALSE, "String"=w1097, "Network Info"=w1098) -> ("error out"=w1091:errorcluster, "TCP Network Connection out"=w1095:refnum<k5>)  [unwired: 6 in]
              n349 = xnode "Read/Write Control"("FPGA VI Reference In"=w1100, "error in"=w1091) -> ("error out"=w1092:errorcluster, "DAQ Cycle Ticks"=w1096:u32)  [unwired: 1 out]
              n350 = call-poly "TCP Write Length and Data.vi"("Error In"=w1092, "Data"=w1096, "connection ID"=w1095) -> ("Error Out"=w1093:errorcluster)  [unwired: 7 in, 1 out]
            }
            frame "Res Mag dI/dt Delay" {
              n351 = call "Command Reply.vi"("Error In"=w1104, "Error?"=FALSE, "String"=w1107, "Network Info"=w1108) -> ("error out"=w1101:errorcluster, "TCP Network Connection out"=w1105:refnum<k5>)  [unwired: 6 in]
              n352 = xnode "Read/Write Control"("FPGA VI Reference In"=w1110, "error in"=w1101) -> ("error out"=w1102:errorcluster, "Res Mag dI/dt Delay"=w1106:u32)  [unwired: 1 out]
              n353 = call-poly "TCP Write Length and Data.vi"("Error In"=w1102, "Data"=w1106, "connection ID"=w1105) -> ("Error Out"=w1103:errorcluster)  [unwired: 7 in, 1 out]
            }
            frame "dI/dT scaling" {
              n354 = call "Command Reply.vi"("Error In"=w1114, "Error?"=FALSE, "String"=w1118, "Network Info"=w1119) -> ("error out"=w1111:errorcluster, "TCP Network Connection out"=w1115:refnum<k5>)  [unwired: 6 in]
              n355 = xnode "Read/Write Control"("FPGA VI Reference In"=w1121, "error in"=w1111) -> ("error out"=w1112:errorcluster, "dI/dT scaling"=w1116:fxp<+/-,35,11>)  [unwired: 1 out]
              n356 = To Double Precision Float(number=w1116) -> (double precision float=w1117:dbl)
              n357 = call-poly "TCP Write Length and Data.vi"("Error In"=w1112, "Data"=w1117, "connection ID"=w1115) -> ("Error Out"=w1113:errorcluster)  [unwired: 7 in, 1 out]
            }
            frame "Cooldown Mode" {
              n358 = call "Command Reply.vi"("Error In"=w1125, "Error?"=FALSE, "String"=w1128, "Network Info"=w1129) -> ("error out"=w1122:errorcluster, "TCP Network Connection out"=w1126:refnum<k5>)  [unwired: 6 in]
              n359 = xnode "Read/Write Control"("FPGA VI Reference In"=w1131, "error in"=w1122) -> ("error out"=w1123:errorcluster, "Cooldown Mode"=w1127:bool)  [unwired: 1 out]
              n360 = call-poly "TCP Write Length and Data.vi"("Error In"=w1123, "Data"=w1127, "connection ID"=w1126) -> ("Error Out"=w1124:errorcluster)  [unwired: 7 in, 1 out]
            }
            frame "Pressure Inlet Limit (BarA)" {
              n361 = call "Command Reply.vi"("Error In"=w1135, "Error?"=FALSE, "String"=w1139, "Network Info"=w1140) -> ("error out"=w1132:errorcluster, "TCP Network Connection out"=w1136:refnum<k5>)  [unwired: 6 in]
              n362 = xnode "Read/Write Control"("FPGA VI Reference In"=w1142, "error in"=w1132) -> ("error out"=w1133:errorcluster, "Pressure Inlet Limit (BarA)"=w1137:fxp<+/-,38,12>)  [unwired: 1 out]
              n363 = To Double Precision Float(number=w1137) -> (double precision float=w1138:dbl)
              n364 = call-poly "TCP Write Length and Data.vi"("Error In"=w1133, "Data"=w1138, "connection ID"=w1136) -> ("Error Out"=w1134:errorcluster)  [unwired: 7 in, 1 out]
            }
            frame "Pressure Outlet Limit (BarA)" {
              n365 = call "Command Reply.vi"("Error In"=w1146, "Error?"=FALSE, "String"=w1150, "Network Info"=w1151) -> ("error out"=w1143:errorcluster, "TCP Network Connection out"=w1147:refnum<k5>)  [unwired: 6 in]
              n366 = xnode "Read/Write Control"("FPGA VI Reference In"=w1153, "error in"=w1143) -> ("error out"=w1144:errorcluster, "Pressure Outlet Limit (BarA)"=w1148:fxp<+/-,38,12>)  [unwired: 1 out]
              n367 = To Double Precision Float(number=w1148) -> (double precision float=w1149:dbl)
              n368 = call-poly "TCP Write Length and Data.vi"("Error In"=w1144, "Data"=w1149, "connection ID"=w1147) -> ("Error Out"=w1145:errorcluster)  [unwired: 7 in, 1 out]
            }
            frame "Pressure Inlet Cooldown Limit" {
              n369 = call "Command Reply.vi"("Error In"=w1157, "Error?"=FALSE, "String"=w1161, "Network Info"=w1162) -> ("error out"=w1154:errorcluster, "TCP Network Connection out"=w1158:refnum<k5>)  [unwired: 6 in]
              n370 = xnode "Read/Write Control"("FPGA VI Reference In"=w1164, "error in"=w1154) -> ("error out"=w1155:errorcluster, "Pressure Inlet Cooldown Limit"=w1159:fxp<+/-,38,12>)  [unwired: 1 out]
              n371 = To Double Precision Float(number=w1159) -> (double precision float=w1160:dbl)
              n372 = call-poly "TCP Write Length and Data.vi"("Error In"=w1155, "Data"=w1160, "connection ID"=w1158) -> ("Error Out"=w1156:errorcluster)  [unwired: 7 in, 1 out]
            }
            frame "Pressure Outlet Cooldown Limit" {
              n373 = call "Command Reply.vi"("Error In"=w1168, "Error?"=FALSE, "String"=w1172, "Network Info"=w1173) -> ("error out"=w1165:errorcluster, "TCP Network Connection out"=w1169:refnum<k5>)  [unwired: 6 in]
              n374 = xnode "Read/Write Control"("FPGA VI Reference In"=w1175, "error in"=w1165) -> ("error out"=w1166:errorcluster, "Pressure Outlet Cooldown Limit"=w1170:fxp<+/-,38,12>)  [unwired: 1 out]
              n375 = To Double Precision Float(number=w1170) -> (double precision float=w1171:dbl)
              n376 = call-poly "TCP Write Length and Data.vi"("Error In"=w1166, "Data"=w1171, "connection ID"=w1169) -> ("Error Out"=w1167:errorcluster)  [unwired: 7 in, 1 out]
            }
            frame "Bore Tube Volt Limit" {
              n377 = call "Command Reply.vi"("Error In"=w1179, "Error?"=FALSE, "String"=w1183, "Network Info"=w1184) -> ("error out"=w1176:errorcluster, "TCP Network Connection out"=w1180:refnum<k5>)  [unwired: 6 in]
              n378 = xnode "Read/Write Control"("FPGA VI Reference In"=w1186, "error in"=w1176) -> ("error out"=w1177:errorcluster, "Bore Tube Volt Limit"=w1181:fxp<+/-,38,12>)  [unwired: 1 out]
              n379 = To Double Precision Float(number=w1181) -> (double precision float=w1182:dbl)
              n380 = call-poly "TCP Write Length and Data.vi"("Error In"=w1177, "Data"=w1182, "connection ID"=w1180) -> ("Error Out"=w1178:errorcluster)  [unwired: 7 in, 1 out]
            }
            frame "Activation Current (kA)" {
              n381 = call "Command Reply.vi"("Error In"=w1190, "Error?"=FALSE, "String"=w1194, "Network Info"=w1195) -> ("error out"=w1187:errorcluster, "TCP Network Connection out"=w1191:refnum<k5>)  [unwired: 6 in]
              n382 = xnode "Read/Write Control"("FPGA VI Reference In"=w1197, "error in"=w1187) -> ("error out"=w1188:errorcluster, "Activation Current (kA)"=w1192:fxp<+/-,38,12>)  [unwired: 1 out]
              n383 = To Double Precision Float(number=w1192) -> (double precision float=w1193:dbl)
              n384 = call-poly "TCP Write Length and Data.vi"("Error In"=w1188, "Data"=w1193, "connection ID"=w1191) -> ("Error Out"=w1189:errorcluster)  [unwired: 7 in, 1 out]
            }
            frame "Ln2 Filter Size" {
              n385 = call "Command Reply.vi"("Error In"=w1201, "Error?"=FALSE, "String"=w1204, "Network Info"=w1205) -> ("error out"=w1198:errorcluster, "TCP Network Connection out"=w1202:refnum<k5>)  [unwired: 6 in]
              n386 = xnode "Read/Write Control"("FPGA VI Reference In"=w1207, "error in"=w1198) -> ("error out"=w1199:errorcluster, "Ln2 Filter Size"=w1203:i16)  [unwired: 1 out]
              n387 = call-poly "TCP Write Length and Data.vi"("Error In"=w1199, "Data"=w1203, "connection ID"=w1202) -> ("Error Out"=w1200:errorcluster)  [unwired: 7 in, 1 out]
            }
            frame "# Consecutive Zeros Fault" {
              n388 = call "Command Reply.vi"("Error In"=w1211, "Error?"=FALSE, "String"=w1214, "Network Info"=w1215) -> ("error out"=w1208:errorcluster, "TCP Network Connection out"=w1212:refnum<k5>)  [unwired: 6 in]
              n389 = xnode "Read/Write Control"("FPGA VI Reference In"=w1217, "error in"=w1208) -> ("error out"=w1209:errorcluster, "# Consecutive Zeros Fault"=w1213:i16)  [unwired: 1 out]
              n390 = call-poly "TCP Write Length and Data.vi"("Error In"=w1209, "Data"=w1213, "connection ID"=w1212) -> ("Error Out"=w1210:errorcluster)  [unwired: 7 in, 1 out]
            }
            frame "Digitize Convert Ticks" {
              n391 = call "Command Reply.vi"("Error In"=w1221, "Error?"=FALSE, "String"=w1224, "Network Info"=w1225) -> ("error out"=w1218:errorcluster, "TCP Network Connection out"=w1222:refnum<k5>)  [unwired: 6 in]
              n392 = xnode "Read/Write Control"("FPGA VI Reference In"=w1227, "error in"=w1218) -> ("error out"=w1219:errorcluster, "Digitize Convert Ticks"=w1223:u32)  [unwired: 1 out]
              n393 = call-poly "TCP Write Length and Data.vi"("Error In"=w1219, "Data"=w1223, "connection ID"=w1222) -> ("Error Out"=w1220:errorcluster)  [unwired: 7 in, 1 out]
            }
            frame "Digitize Reset Ticks" {
              n394 = call "Command Reply.vi"("Error In"=w1231, "Error?"=FALSE, "String"=w1234, "Network Info"=w1235) -> ("error out"=w1228:errorcluster, "TCP Network Connection out"=w1232:refnum<k5>)  [unwired: 6 in]
              n395 = xnode "Read/Write Control"("FPGA VI Reference In"=w1237, "error in"=w1228) -> ("error out"=w1229:errorcluster, "Digitize Reset Ticks"=w1233:u32)  [unwired: 1 out]
              n396 = call-poly "TCP Write Length and Data.vi"("Error In"=w1229, "Data"=w1233, "connection ID"=w1232) -> ("Error Out"=w1230:errorcluster)  [unwired: 7 in, 1 out]
            }
            frame "Convert Clock Ticks" {
              n397 = call "Command Reply.vi"("Error In"=w1241, "Error?"=FALSE, "String"=w1244, "Network Info"=w1245) -> ("error out"=w1238:errorcluster, "TCP Network Connection out"=w1242:refnum<k5>)  [unwired: 6 in]
              n398 = xnode "Read/Write Control"("FPGA VI Reference In"=w1247, "error in"=w1238) -> ("error out"=w1239:errorcluster, "Convert Clock Ticks"=w1243:u32)  [unwired: 1 out]
              n399 = call-poly "TCP Write Length and Data.vi"("Error In"=w1239, "Data"=w1243, "connection ID"=w1242) -> ("Error Out"=w1240:errorcluster)  [unwired: 7 in, 1 out]
            }
            frame "Digitize Read Delay Ticks" {
              n400 = call "Command Reply.vi"("Error In"=w1251, "Error?"=FALSE, "String"=w1254, "Network Info"=w1255) -> ("error out"=w1248:errorcluster, "TCP Network Connection out"=w1252:refnum<k5>)  [unwired: 6 in]
              n401 = xnode "Read/Write Control"("FPGA VI Reference In"=w1257, "error in"=w1248) -> ("error out"=w1249:errorcluster, "Digitize Read Delay Ticks"=w1253:u32)  [unwired: 1 out]
              n402 = call-poly "TCP Write Length and Data.vi"("Error In"=w1249, "Data"=w1253, "connection ID"=w1252) -> ("Error Out"=w1250:errorcluster)  [unwired: 7 in, 1 out]
            }
            frame "Digitize # Bits" {
              n403 = call "Command Reply.vi"("Error In"=w1261, "Error?"=FALSE, "String"=w1264, "Network Info"=w1265) -> ("error out"=w1258:errorcluster, "TCP Network Connection out"=w1262:refnum<k5>)  [unwired: 6 in]
              n404 = xnode "Read/Write Control"("FPGA VI Reference In"=w1267, "error in"=w1258) -> ("error out"=w1259:errorcluster, "Digitize # Bits"=w1263:u32)  [unwired: 1 out]
              n405 = call-poly "TCP Write Length and Data.vi"("Error In"=w1259, "Data"=w1263, "connection ID"=w1262) -> ("Error Out"=w1260:errorcluster)  [unwired: 7 in, 1 out]
            }
            frame "Magnet Configuration Data" {
              n406 = call "Command Reply.vi"("Error In"=w1274, "Error?"=FALSE, "String"=w1276, "Network Info"=w1277) -> ("error out"=w1272:errorcluster, "TCP Network Connection out"=w1275:refnum<k5>)  [unwired: 6 in]
              n407 = xnode "Read/Write Control"("FPGA VI Reference In"=w1279, "error in"=w1272) -> ("error out"=w1270:errorcluster, "Magnet Configuration Data"=w1271:T8)  [unwired: 1 out]
              n408 = Flatten To String(anything=w1271, error in (no error)=w1270) -> (data string=w1268:string, error out=w1269:errorcluster)  [unwired: 2 in, 1 out]
              n409 = call-poly "TCP Write Length and Data.vi"("Error In"=w1269, "Data"=w1268, "connection ID"=w1275) -> ("Error Out"=w1273:errorcluster)  [unwired: 7 in, 1 out]
            }
            frame "Signal Injection On" {
              n410 = call "Command Reply.vi"("Error In"=w1285, "Error?"=FALSE, "String"=w1287, "Network Info"=w1288) -> ("error out"=w1282:errorcluster, "TCP Network Connection out"=w1286:refnum<k5>)  [unwired: 6 in]
              n411 = xnode "Read/Write Control"("FPGA VI Reference In"=w1283, "error in"=w1282) -> ("error out"=w1281:errorcluster, "Signal Injection On"=w1280:bool)  [unwired: 1 out]
              n412 = call-poly "TCP Write Length and Data.vi"("Error In"=w1281, "Data"=w1280, "connection ID"=w1286) -> ("Error Out"=w1284:errorcluster)  [unwired: 7 in, 1 out]
            }
            frame "Inject Frequency (Hz)" {
              n413 = call "Command Reply.vi"("Error In"=w1293, "Error?"=FALSE, "String"=w1297, "Network Info"=w1298) -> ("error out"=w1290:errorcluster, "TCP Network Connection out"=w1294:refnum<k5>)  [unwired: 6 in]
              n414 = xnode "Read/Write Control"("FPGA VI Reference In"=w1300, "error in"=w1290) -> ("error out"=w1291:errorcluster, "Inject frequency (Hz)"=w1295:fxp<+,32,16>)  [unwired: 1 out]
              n415 = To Double Precision Float(number=w1295) -> (double precision float=w1296:dbl)
              n416 = call-poly "TCP Write Length and Data.vi"("Error In"=w1291, "Data"=w1296, "connection ID"=w1294) -> ("Error Out"=w1292:errorcluster)  [unwired: 7 in, 1 out]
            }
            frame "Inject Offset" {
              n417 = call "Command Reply.vi"("Error In"=w1304, "Error?"=FALSE, "String"=w1308, "Network Info"=w1309) -> ("error out"=w1301:errorcluster, "TCP Network Connection out"=w1305:refnum<k5>)  [unwired: 6 in]
              n418 = xnode "Read/Write Control"("FPGA VI Reference In"=w1311, "error in"=w1301) -> ("error out"=w1302:errorcluster, "Inject Offset"=w1306:fxp<+/-,16,5>)  [unwired: 1 out]
              n419 = To Double Precision Float(number=w1306) -> (double precision float=w1307:dbl)
              n420 = call-poly "TCP Write Length and Data.vi"("Error In"=w1302, "Data"=w1307, "connection ID"=w1305) -> ("Error Out"=w1303:errorcluster)  [unwired: 7 in, 1 out]
            }
            frame "Inject Channel" {
              n421 = call "Command Reply.vi"("Error In"=w1315, "Error?"=FALSE, "String"=w1318, "Network Info"=w1319) -> ("error out"=w1312:errorcluster, "TCP Network Connection out"=w1316:refnum<k5>)  [unwired: 6 in]
              n422 = xnode "Read/Write Control"("FPGA VI Reference In"=w1321, "error in"=w1312) -> ("error out"=w1313:errorcluster, "Inject Channel"=w1317:i32)  [unwired: 1 out]
              n423 = call-poly "TCP Write Length and Data.vi"("Error In"=w1313, "Data"=w1317, "connection ID"=w1316) -> ("Error Out"=w1314:errorcluster)  [unwired: 7 in, 1 out]
            }
            frame "Scale" {
              n424 = call "Command Reply.vi"("Error In"=w1325, "Error?"=FALSE, "String"=w1328, "Network Info"=w1329) -> ("error out"=w1322:errorcluster, "TCP Network Connection out"=w1326:refnum<k5>)  [unwired: 6 in]
              n425 = xnode "Read/Write Control"("FPGA VI Reference In"=w1331, "error in"=w1322) -> ("error out"=w1323:errorcluster, "Scale"=w1327:i16[])  [unwired: 1 out]
              n426 = call-poly "TCP Write Length and Data.vi"("Error In"=w1323, "Data"=w1327, "connection ID"=w1326) -> ("Error Out"=w1324:errorcluster)  [unwired: 7 in, 1 out]
            }
            frame "Offset" {
              n427 = call "Command Reply.vi"("Error In"=w1335, "Error?"=FALSE, "String"=w1338, "Network Info"=w1339) -> ("error out"=w1332:errorcluster, "TCP Network Connection out"=w1336:refnum<k5>)  [unwired: 6 in]
              n428 = xnode "Read/Write Control"("FPGA VI Reference In"=w1341, "error in"=w1332) -> ("error out"=w1333:errorcluster, "Offset"=w1337:i16[])  [unwired: 1 out]
              n429 = call-poly "TCP Write Length and Data.vi"("Error In"=w1333, "Data"=w1337, "connection ID"=w1336) -> ("Error Out"=w1334:errorcluster)  [unwired: 7 in, 1 out]
            }
            frame "Low Current (kA)" {
              n430 = call "Command Reply.vi"("Error In"=w1346, "Error?"=FALSE, "String"=w1349, "Network Info"=w1350) -> ("error out"=w1343:errorcluster, "TCP Network Connection out"=w1347:refnum<k5>)  [unwired: 6 in]
              n431 = xnode "Read/Write Control"("FPGA VI Reference In"=w1352, "error in"=w1343) -> ("error out"=w1344:errorcluster, "Low Current (kA)"=w1348:fxp<+/-,38,12>)  [unwired: 1 out]
              n432 = To Double Precision Float(number=w1348) -> (double precision float=w1342:dbl)
              n433 = call-poly "TCP Write Length and Data.vi"("Error In"=w1344, "Data"=w1342, "connection ID"=w1347) -> ("Error Out"=w1345:errorcluster)  [unwired: 7 in, 1 out]
            }
            frame "Low Current Ticks" {
              n434 = call "Command Reply.vi"("Error In"=w1356, "Error?"=FALSE, "String"=w1359, "Network Info"=w1360) -> ("error out"=w1353:errorcluster, "TCP Network Connection out"=w1357:refnum<k5>)  [unwired: 6 in]
              n435 = xnode "Read/Write Control"("FPGA VI Reference In"=w1362, "error in"=w1353) -> ("error out"=w1354:errorcluster, "Low Current Ticks"=w1358:u32)  [unwired: 1 out]
              n436 = call-poly "TCP Write Length and Data.vi"("Error In"=w1354, "Data"=w1358, "connection ID"=w1357) -> ("Error Out"=w1355:errorcluster)  [unwired: 7 in, 1 out]
            }
            frame "Ticks to Close Relief" {
              n437 = call "Command Reply.vi"("Error In"=w1366, "Error?"=FALSE, "String"=w1369, "Network Info"=w1370) -> ("error out"=w1363:errorcluster, "TCP Network Connection out"=w1367:refnum<k5>)  [unwired: 6 in]
              n438 = xnode "Read/Write Control"("FPGA VI Reference In"=w1372, "error in"=w1363) -> ("error out"=w1364:errorcluster, "Ticks to Close Relief"=w1368:u32)  [unwired: 1 out]
              n439 = call-poly "TCP Write Length and Data.vi"("Error In"=w1364, "Data"=w1368, "connection ID"=w1367) -> ("Error Out"=w1365:errorcluster)  [unwired: 7 in, 1 out]
            }
            frame "Delay Ticks Between Bkr Reset" {
              n440 = call "Command Reply.vi"("Error In"=w1376, "Error?"=FALSE, "String"=w1379, "Network Info"=w1380) -> ("error out"=w1373:errorcluster, "TCP Network Connection out"=w1377:refnum<k5>)  [unwired: 6 in]
              n441 = xnode "Read/Write Control"("FPGA VI Reference In"=w1382, "error in"=w1373) -> ("error out"=w1374:errorcluster, "Delay Ticks Between Bkr Reset"=w1378:u32)  [unwired: 1 out]
              n442 = call-poly "TCP Write Length and Data.vi"("Error In"=w1374, "Data"=w1378, "connection ID"=w1377) -> ("Error Out"=w1375:errorcluster)  [unwired: 7 in, 1 out]
            }
            frame "Breaker Reset Ticks" {
              n443 = call "Command Reply.vi"("Error In"=w1386, "Error?"=FALSE, "String"=w1389, "Network Info"=w1390) -> ("error out"=w1383:errorcluster, "TCP Network Connection out"=w1387:refnum<k5>)  [unwired: 6 in]
              n444 = xnode "Read/Write Control"("FPGA VI Reference In"=w1392, "error in"=w1383) -> ("error out"=w1384:errorcluster, "Breaker Reset Ticks"=w1388:u32)  [unwired: 1 out]
              n445 = call-poly "TCP Write Length and Data.vi"("Error In"=w1384, "Data"=w1388, "connection ID"=w1387) -> ("Error Out"=w1385:errorcluster)  [unwired: 7 in, 1 out]
            }
            frame "PS Enable Reset Ticks" {
              n446 = call "Command Reply.vi"("Error In"=w1396, "Error?"=FALSE, "String"=w1399, "Network Info"=w1400) -> ("error out"=w1393:errorcluster, "TCP Network Connection out"=w1397:refnum<k5>)  [unwired: 6 in]
              n447 = xnode "Read/Write Control"("FPGA VI Reference In"=w1402, "error in"=w1393) -> ("error out"=w1394:errorcluster, "PS Enable Reset Ticks"=w1398:u32)  [unwired: 1 out]
              n448 = call-poly "TCP Write Length and Data.vi"("Error In"=w1394, "Data"=w1398, "connection ID"=w1397) -> ("Error Out"=w1395:errorcluster)  [unwired: 7 in, 1 out]
            }
            frame "Reset Digitizer Ticks" {
              n449 = call "Command Reply.vi"("Error In"=w1406, "Error?"=FALSE, "String"=w1409, "Network Info"=w1410) -> ("error out"=w1403:errorcluster, "TCP Network Connection out"=w1407:refnum<k5>)  [unwired: 6 in]
              n450 = xnode "Read/Write Control"("FPGA VI Reference In"=w1412, "error in"=w1403) -> ("error out"=w1404:errorcluster, "Reset Digitizer Ticks"=w1408:u32)  [unwired: 1 out]
              n451 = call-poly "TCP Write Length and Data.vi"("Error In"=w1404, "Data"=w1408, "connection ID"=w1407) -> ("Error Out"=w1405:errorcluster)  [unwired: 7 in, 1 out]
            }
            frame "Low Current Delay Factor" {
              n452 = call "Command Reply.vi"("Error In"=w1416, "Error?"=FALSE, "String"=w1419, "Network Info"=w1420) -> ("error out"=w1413:errorcluster, "TCP Network Connection out"=w1417:refnum<k5>)  [unwired: 6 in]
              n453 = xnode "Read/Write Control"("FPGA VI Reference In"=w1422, "error in"=w1413) -> ("error out"=w1414:errorcluster, "Low Current Delay Factor"=w1418:u16)  [unwired: 1 out]
              n454 = call-poly "TCP Write Length and Data.vi"("Error In"=w1414, "Data"=w1418, "connection ID"=w1417) -> ("Error Out"=w1415:errorcluster)  [unwired: 7 in, 1 out]
            }
            frame "Data Size" {
              n455 = call "Command Reply.vi"("Error In"=w1426, "Error?"=FALSE, "String"=w1428, "Network Info"=w1429) -> ("error out"=w1424:errorcluster, "TCP Network Connection out"=w1427:refnum<k5>)  [unwired: 6 in]
              n456 = global read "RT Host Globals.vi" "Data Size"() -> (w1423:u32)
              n457 = call-poly "TCP Write Length and Data.vi"("Error In"=w1424, "Data"=w1423, "connection ID"=w1427) -> ("Error Out"=w1425:errorcluster)  [unwired: 7 in, 1 out]
            }
            frame "Data Period" {
              n458 = call "Command Reply.vi"("Error In"=w1436, "Error?"=FALSE, "String"=w1438, "Network Info"=w1439) -> ("error out"=w1434:errorcluster, "TCP Network Connection out"=w1437:refnum<k5>)  [unwired: 6 in]
              n459 = global read "RT Host Globals.vi" "Decimation Factor"() -> (w1433:u32)
              n460 = global read "RT Host Globals.vi" "Raw Data Period"() -> (w1432:dbl)
              n461 = Multiply(x=w1433, y=w1432) -> (x*y=w1431:dbl)
              n462 = call-poly "TCP Write Length and Data.vi"("Error In"=w1434, "Data"=w1431, "connection ID"=w1437) -> ("Error Out"=w1435:errorcluster)  [unwired: 7 in, 1 out]
            }
            frame "Version FPGA" {
              n463 = call "Command Reply.vi"("Error In"=w1451, "Error?"=FALSE, "String"=w1453, "Network Info"=w1454) -> ("error out"=w1444:errorcluster, "TCP Network Connection out"=w1452:refnum<k5>)  [unwired: 6 in]
              n464 = xnode "Read/Write Control"("FPGA VI Reference In"=w1449, "error in"=w1444) -> ("error out"=w1443:errorcluster, "Major"=w1448:u8, "Minor"=w1447:u8, "Fix"=w1446:u8, "Build"=w1445:u8)  [unwired: 1 out]
              n465 = Format Into String(format string="%d.%d.%d.%d", w1448, w1447, w1446, w1445) -> (resulting string=w1441:string)  [unwired: 2 in, 1 out]
              n466 = call-poly "TCP Write Length and Data.vi"("Error In"=w1443, "Data"=w1441, "connection ID"=w1452) -> ("Error Out"=w1450:errorcluster)  [unwired: 7 in, 1 out]
            }
            frame "Version RT System" {
              n467 = global read "RT Host Globals.vi" "Minor"() -> (w1459:u8)
              n468 = global read "RT Host Globals.vi" "Major"() -> (w1460:u8)
              n469 = global read "RT Host Globals.vi" "Build"() -> (w1456:u8)
              n470 = global read "RT Host Globals.vi" "Fix"() -> (w1458:u8)
              n471 = Format Into String(format string="%d.%d.%d.%d", w1460, w1459, w1458, w1456) -> (resulting string=w1461:string)  [unwired: 2 in, 1 out]
              n472 = call "Command Reply.vi"("Error In"=w1464, "Error?"=FALSE, "String"=w1466, "Network Info"=w1467) -> ("error out"=w1457:errorcluster, "TCP Network Connection out"=w1465:refnum<k5>)  [unwired: 6 in]
              n473 = call-poly "TCP Write Length and Data.vi"("Error In"=w1457, "Data"=w1461, "connection ID"=w1465) -> ("Error Out"=w1463:errorcluster)  [unwired: 7 in, 1 out]
            }
            frame "Start DateStamp" {
              n474 = global read "RT Host Globals.vi" "Start DateStamp"() -> (w1469:timestamp)
              n475 = call "Command Reply.vi"("Error In"=w1472, "Error?"=FALSE, "String"=w1474, "Network Info"=w1475) -> ("error out"=w1470:errorcluster, "TCP Network Connection out"=w1473:refnum<k5>)  [unwired: 6 in]
              n476 = call-poly "TCP Write Length and Data.vi"("Error In"=w1470, "Data"=w1469, "connection ID"=w1473) -> ("Error Out"=w1471:errorcluster)  [unwired: 7 in, 1 out]
            }
            frame "Calibration DateStamp" {
              n477 = global read "RT Host Globals.vi" "Calibration DateStamp"() -> (w1477:timestamp)
              n478 = call "Command Reply.vi"("Error In"=w1480, "Error?"=FALSE, "String"=w1482, "Network Info"=w1483) -> ("error out"=w1478:errorcluster, "TCP Network Connection out"=w1481:refnum<k5>)  [unwired: 6 in]
              n479 = call-poly "TCP Write Length and Data.vi"("Error In"=w1478, "Data"=w1477, "connection ID"=w1481) -> ("Error Out"=w1479:errorcluster)  [unwired: 7 in, 1 out]
            }
            frame "Notification Email" {
              n480 = global read "RT Host Globals.vi" "Notification Email"() -> (w1485:string)
              n481 = call "Command Reply.vi"("Error In"=w1488, "Error?"=FALSE, "String"=w1490, "Network Info"=w1491) -> ("error out"=w1486:errorcluster, "TCP Network Connection out"=w1489:refnum<k5>)  [unwired: 6 in]
              n482 = call-poly "TCP Write Length and Data.vi"("Error In"=w1486, "Data"=w1485, "connection ID"=w1489) -> ("Error Out"=w1487:errorcluster)  [unwired: 7 in, 1 out]
            }
          }
        }
        frame "LISTFILES" {
          # "List Stored Trip Files"
          n483 = call "Get Shared Data Dir.vi"() -> ("Error Out"=w1509:errorcluster, "Data Directory Path"=w1496:path)  [unwired: 2 in]
          n484 = call "Command Reply.vi"("Error In"=w1505, "Error?"=FALSE, "String"=w1503, "Network Info"=w1500) -> ("error out"=w1504:errorcluster, "TCP Network Connection out"=w1501:refnum<k5>)  [unwired: 6 in]
          n485 = Merge Errors(w1509, w1504) -> (w1508:errorcluster)
          n486 = List Folder(path=w1496, pattern="SCH Log *", error in=w1508) -> (path out=w1493:path, filenames=w1507:string[], error out=w1495:errorcluster)  [unwired: 1 in, 1 out]
          n487 = List Folder(path=w1493, pattern="SCH Trip *", error in=w1495) -> (filenames=w1497:string[], error out=w1494:errorcluster)  [unwired: 1 in, 2 out]
          n488 = Build Array (concatenate)(w1507, w1497) -> (w1498:string[])
          n489 = call-poly "TCP Write Length and Data.vi"("Error In"=w1494, "Data"=w1498, "connection ID"=w1501) -> ("Error Out"=w1506:errorcluster)  [unwired: 7 in, 1 out]
        }
        frame "DOWNLOAD" {
          # "Download Stored Trip File"
          n490 = call "Command Reply.vi"("Error In"=w1518, "Error?"=FALSE, "String"=w1513, "Network Info"=w1511) -> ("error out"=w1517:errorcluster, "TCP Network Connection out"=w1512:refnum<k5>)  [unwired: 6 in]
          n491 = call "Download Stored Trip File.vi"("error in (no error)"=w1517, "File Name"=w1514, "TCP Network Connection in"=w1512) -> ("error out"=w1515:errorcluster)  [unwired: 8 in]
        }
        frame "PASSWORD" {
          # "Challenge and Response Password"
          n492 = call "Command Reply.vi"("Error In"=w1532, "Error?"=FALSE, "String"=w1529, "Network Info"=w1527) -> ("error out"=w1531:errorcluster, "TCP Network Connection out"=w1528:refnum<k5>)  [unwired: 6 in]
          n493 = call "Check Password.vi"("error in (no error)"=w1531, "TCP Network Connection in"=w1528) -> ("error out"=w1524:errorcluster, "Authorized Level"=w1526:enum16{"Read Only", "Operator", "Admin"}, "connection ID out"=w1521:refnum<k5>)  [unwired: 7 in]
          n494 = Greater?(x=w1526, y=RT_System_Auth_Level."Read Only" ("Authorized")) -> (0:w1522:bool)
          n495 = case shown="True" w1522 {
            tunnel: w1526 -> [w1534 w1535]
            tunnel: [w1534 w1535] -> w1525
            tunnel: w1524 -> [w1533 w1537]
            tunnel: [w1533 w1536] -> w1523
            tunnel: w1521 -> [_ w1538]
            frame False {
            }
            frame True {
              n496 = call-poly "TCP Write Length and Data.vi"("Error In"=w1537, "Data"=w1535, "connection ID"=w1538) -> ("Error Out"=w1536:errorcluster)  [unwired: 7 in, 1 out]
            }
          }
          n497 = Bundle By Name(cluster=w1527, "Authorized"=w1525) -> (w1519:T1)
        }
      }
    }
    frame Error {
      # "Network Conneciton ID Invalid"
      # "Network Read Timeout"
      # "Network Connection Closed"
      n498 = call <vilib>:"Clear Errors.vi"("error in (no error)"=w1545, "specific error code to clear (0: all)"=56) -> ("error out"=w1541:errorcluster)  [unwired: 4 in, 1 out]
      n499 = call "System Reporting.vi"("Error In"=w1541) -> ()  [unwired: 9 in, 2 out]
      n500 = call <vilib>:"Clear Errors.vi"("error in (no error)"=w1541, "specific error code to clear (0: all)"=1) -> ("error out"=w1542:errorcluster, "specific error cleared?"=w1539:bool)  [unwired: 4 in]
      n501 = call <vilib>:"Clear Errors.vi"("error in (no error)"=w1542, "specific error code to clear (0: all)"=66) -> ("error out"=w1548:errorcluster, "specific error cleared?"=w1544:bool)  [unwired: 4 in]
      n502 = Or(x=w1539, y=w1544) -> (x .or. y?=w1540:bool)
    }
  }
  "Error Out" <- w13
  "Network Info out" <- w7
  n503 = flat-sequence {
    tunnel: w7 -> [w1551]
    tunnel: [w1550] -> w2
    frame #0 {
      n504 = Unbundle By Name(w1551) -> ("Last Comm Time"=w1552:timestamp)
      n505 = Get Date/Time In Seconds() -> (seconds since 1Jan1904=w1553:timestamp)
      n506 = Subtract(x=w1553, y=w1552) -> (x-y=w1550:dbl)
    }
  }
  n507 = global read "RT Host Globals.vi" "Sec Drop Connection"() -> (w8:dbl)
  n508 = Greater?(x=w2, y=w8) -> (0:w6:bool)
  n509 = disable-structure shown="DEBUG==TRUE" {
    disable-tunnel: w2 -> [_ w1556]
    frame condition #0 (active) {
    }
    frame condition #1 {
      n510 = Greater?(x=w1556, y=10.0) -> (0:w1554:bool)
      n511 = case shown="True" w1554 {
        tunnel: w1556 -> [_ w1557]
        frame False {
        }
        frame True {
          n512 = Format Into String(format string="Dormant Time %.1f", w1557) -> (resulting string=w1558:string)  [unwired: 2 in, 1 out]
          n513 = call "System Reporting.vi"("String"=w1558) -> ()  [unwired: 9 in, 2 out]
        }
      }
    }
  }
  n514 = Or(x=w6, y=w4) -> (x .or. y?=→"Connection Dormant":bool)
